vi "PJ1_ui-commu_1 -test.vi"() -> ()   [LabVIEW 2024]
uses:
  <vilib>/express/express analysis/Spectral/XNode/ExpressSpectralMeasurementsBlockNode.xnode
  <vilib>/express/express analysis/Spectral/Block/exnSpectralBlock spectral measurements PSD poly.vi
  <vilib>/express/express analysis/Spectral/Block/exnSpectralBlock spectral measurements PSD DDT.vi
  contron/Control 6.ctl
  contron/Control 7.ctl
  contron/Control 8.ctl
  <vilib>/picture/picture.llb/imagedata.ctl
  contol_vr 23/Control 9.ctl
  contol_vr 23/Control 3.ctl
  contol_vr 23/Control 4.ctl
  contol_vr 23/6.ctl
  contol_vr 23/66.ctl
  contron/Control 5.ctl
panel:
  out "Clear4":bool
  out "Clear 3":bool
  out "Clear2":bool
  out "check":bool
  out "Clear1":bool
  out "com":bool
  out "call":bool
  out "ele":bool
  in  "Baseline":bool
  out "555":bool
  out "6 HZ 2":bool
  out "image data":T1
  out "7 HZ":bool
  in  "Upper Cut-Off":dbl=40.0
  out "PSD":dynamicdata(graph)
  out "PSD MAX":dbl
  out "Index ที่มากที่สุด":i32
  out "max value":dbl
  out "B 18+1":dbl
  out "N 18+1":dbl
  in  "Aj 18+1":dbl
  out "B 18+1":dbl
  out "PSD 18+1":dbl
  out "B 18":dbl
  out "N 18":dbl
  in  "Aj 18":dbl
  out "B 18":dbl
  out "PSD 18":dbl
  out "B 18-1":dbl
  out "N 18-1":dbl
  in  "Aj 18-1":dbl
  out "B 18-1":dbl
  out "PSD 18-1":dbl
  out "9 Hz":dbl[](array[numeric])
  out "Max Index 9":i32
  out "PSD max 9":dbl
  out "PSD 9-1":dbl
  out "B 9-1":dbl
  in  "Aj 9-1":dbl
  out "N 9-1":dbl
  out "B 9-1":dbl
  out "PSD 9":dbl
  out "B 9":dbl
  in  "Aj 9":dbl
  out "N 9":dbl
  out "B 9":dbl
  out "PSD 9+1":dbl
  out "B 9+1":dbl
  in  "Aj 9+1":dbl
  out "N 9+1":dbl
  out "B 9+1":dbl
  out "8 Hz":dbl[](array[numeric])
  out "Max Index 8":i32
  out "PSD max 8":dbl
  out "B 16+1":dbl
  out "N 16+1":dbl
  in  "Aj  16+1":dbl
  out "B 16+1":dbl
  out "PSD  16+1":dbl
  out "B 16":dbl
  out "N  16":dbl
  in  "Aj  16":dbl
  out "B 16":dbl
  out "PSD  16":dbl
  out "B 16-1":dbl
  out "N  16-1":dbl
  in  "Aj   16-1":dbl
  out "B   16-1":dbl
  out "PSD 16-1":dbl
  out "B 8+1":dbl
  out "N 8+1":dbl
  in  "Aj  8+1":dbl
  out "B  8+1":dbl
  out "PSD 8+1":dbl
  out "B 8":dbl
  out "N  8":dbl
  in  "Aj  8":dbl
  out "B  8":dbl
  out "PSD 8":dbl
  out "B 8-1":dbl
  out "N  8-1":dbl
  in  "Aj  8-1":dbl
  out "B  8-1":dbl
  out "PSD 8-1":dbl
  out "PSD 14+1":dbl
  out "B 14+1":dbl
  in  "Aj 14+1":dbl
  out "N 14+1":dbl
  out "B 14+1":dbl
  out "PSD 14":dbl
  out "B 14":dbl
  in  "Aj 14":dbl
  out "N 14":dbl
  out "B 14":dbl
  out "PSD 14-1":dbl
  out "B 14-1":dbl
  in  "Aj 14-1":dbl
  out "N 14-1":dbl
  out "B 14-1":dbl
  out "PSD7+1":dbl
  out "B7+1":dbl
  in  "Aj7+1":dbl
  out "N7+1":dbl
  out "B7+1":dbl
  out "PSD 7":dbl
  out "B 7":dbl
  in  "Aj 7":dbl
  out "N7":dbl
  out "B7":dbl
  out "7 Hz":dbl[](array[numeric])
  out "Max Index 7":i32
  out "PSD max 7":dbl
  out "PSD 7-1":dbl
  out "B 7-1":dbl
  in  "Aj 7-1":dbl
  out "N7-1":dbl
  out "B7-1":dbl
  out "B12-1":dbl
  out "N12-1":dbl
  in  "Aj 12-1":dbl
  out "B 12-1":dbl
  out "PSD 12-1":dbl
  out "B12":dbl
  out "N12":dbl
  in  "Aj 12":dbl
  out "B12":dbl
  out "PSD 12":dbl
  out "B12+1":dbl
  out "N12+1":dbl
  in  "Aj 12+1":dbl
  out "B 12+1":dbl
  out "PSD 12+1":dbl
  out "B6+1":dbl
  out "N6+1":dbl
  in  "Aj 6+1":dbl
  out "B 6+1":dbl
  out "PSD 6+1":dbl
  out "B6":dbl
  out "N6":dbl
  in  "Aj 6":dbl
  out "B6":dbl
  out "PSD 6":dbl
  out "PSD 6-1":dbl
  out "6 Hz":dbl[](array[numeric])
  out "Max Index 6":i32
  out "PSD max 6":dbl
  out "B 6-1":dbl
  in  "Aj 6-1":dbl
  out "N6-1":dbl
  out "B6-1":dbl
  out "appended array":dbl[][](array[numeric])
  out "Filtered Signal":dynamicdata(graph)
  in  "Lower Cut-Off":dbl=1.0
  out "data":dynamicdata(graph) caption="Raw Data"
  in  "number of samples":i32=1000
  in  "rate":dbl=200.0 min=200.0 max=200.0
  out "?":bool
  out "?":bool
  out "?":bool
  out "?":bool
  out "?":bool
  out "?":bool
  out "?":bool
  out "?":bool
  out "?":bool
  out "?":bool
  out "?":bool=TRUE
  out "?":bool=TRUE
  out "?":bool=TRUE
  out "?":bool=TRUE
  out "?":bool=TRUE
  out "?":bool=TRUE
  out "?":bool=TRUE
  out "?":bool=TRUE
  out "?":bool=TRUE
  out "?":bool=TRUE
  out "?":bool
  out "?":bool
  out "?":bool
  out "?":bool
  out "?":bool
  out "?":bool
  out "?":bool
  out "?":bool
  out "?":bool
  out "?":bool
  out "?":bool=TRUE
  out "?":bool=TRUE
  out "?":bool=TRUE
  out "?":bool=TRUE
  out "?":bool=TRUE
  out "?":bool=TRUE
  out "?":bool=TRUE
  out "?":bool=TRUE
  out "?":bool=TRUE
  out "?":bool=TRUE
  out "?":bool
  out "?":bool
  out "?":bool
  out "?":bool
  out "?":bool
  out "?":bool
  out "?":bool
  out "?":bool
  out "?":bool
  out "?":bool
  out "?":bool=TRUE
  out "?":bool=TRUE
  out "?":bool=TRUE
  out "?":bool=TRUE
  out "?":bool=TRUE
  out "?":bool=TRUE
  out "?":bool=TRUE
  out "?":bool=TRUE
  out "?":bool=TRUE
  out "?":bool=TRUE
  out "?":bool
  out "?":bool
  out "?":bool
  out "?":bool
  out "?":bool
  out "?":bool
  out "?":bool
  out "?":bool
  out "?":bool
  out "?":bool
  out "?":bool=TRUE
  out "?":bool=TRUE
  out "?":bool=TRUE
  out "?":bool=TRUE
  out "?":bool=TRUE
  out "?":bool=TRUE
  out "?":bool=TRUE
  out "?":bool=TRUE
  out "?":bool=TRUE
  out "?":bool=TRUE
  out "9 HZ":bool
  out "8 HZ":bool
  in  "Tab Control":T2(tab)
  out "Emotion 7":bool
  out "Emotion 6":bool
  out "Emotion 5":bool
  out "Emotion 4":bool
  out "ele":T3
  out "Emer":bool
  out "call":T4
  out "commu":T5
  out "Activity":bool
  out "8-2":bool
  out "cummu_back":bool
  out "cummu_2":bool
  out "cummu_1":bool
  out "Emotion":bool
  out "ACC":T6
  out "back_page2":T7
  in  "send":bool
  out "call_back":bool
  out "call_3":bool
  out "call_back":bool
  out "call_2":bool
  out "call_1":bool
  out "1 3":bool
  out "1 2":T8
  out "1":bool
  out "String 2":string
  in  "SOS CALLING":bool
  in  "Search Button 2":bool
  out "ele_back":bool
  out "ele_3":bool
  out "ele_2":bool
  out "ele_1":bool
  out "ele_2":bool
  out "ele_3":bool
  out "ele_1":bool
  out "BACK_Page4":bool
  out "BACK_page5":bool
  out "Emotion 3":bool
  out "Emotion 2":bool
  in  "BACK_Page5":bool=TRUE
  in  "Button 3":bool=TRUE
  in  "Button 2":bool=TRUE
  in  "Button 1":bool=TRUE
  out "Emotion 1":bool
  out "Emotion 11":bool
  in  "BACK_Page6":T9
  out "Emotion 10":bool
  out "Emotion 9":bool
  out "Emotion 8":bool
  in  "Activity 1":path
  out "new picture":picture
  in  "Activity 2":path
  in  "Activity 3":path
  out "new picture 2":picture
  out "new picture 3":picture
  out "Emotion 19":bool
  out "Emotion 18":bool
  out "Emotion 17":bool
  out "Emotion 16":bool
  out "new picture 7":picture
  in  "AAC13":path
  in  "Massage Send 3":string
  out "new picture 6":picture
  in  "AAC1 2":path
  in  "Massage Send 2":string
  out "new picture 5":picture
  in  "AAC1":path
  in  "BACK_Page7":bool
  in  "Massage Send 2":string
  out "Message Display":string
  in  "send 3":bool
  in  "Message Send":string
  in  "Clearpage 2":bool
  in  "Text3":T10
  in  "Text2":T11
  in  "Text1":bool
  in  "send 2":bool
  # "MENU"
  # "COMMUNICATION"
  # "SOS CALLING"
  # "Tel."
  # "ELECTRICAL DEVICES"
  # "EMOTIONS"
  # "ACTIVITIES"
  # "AAC"
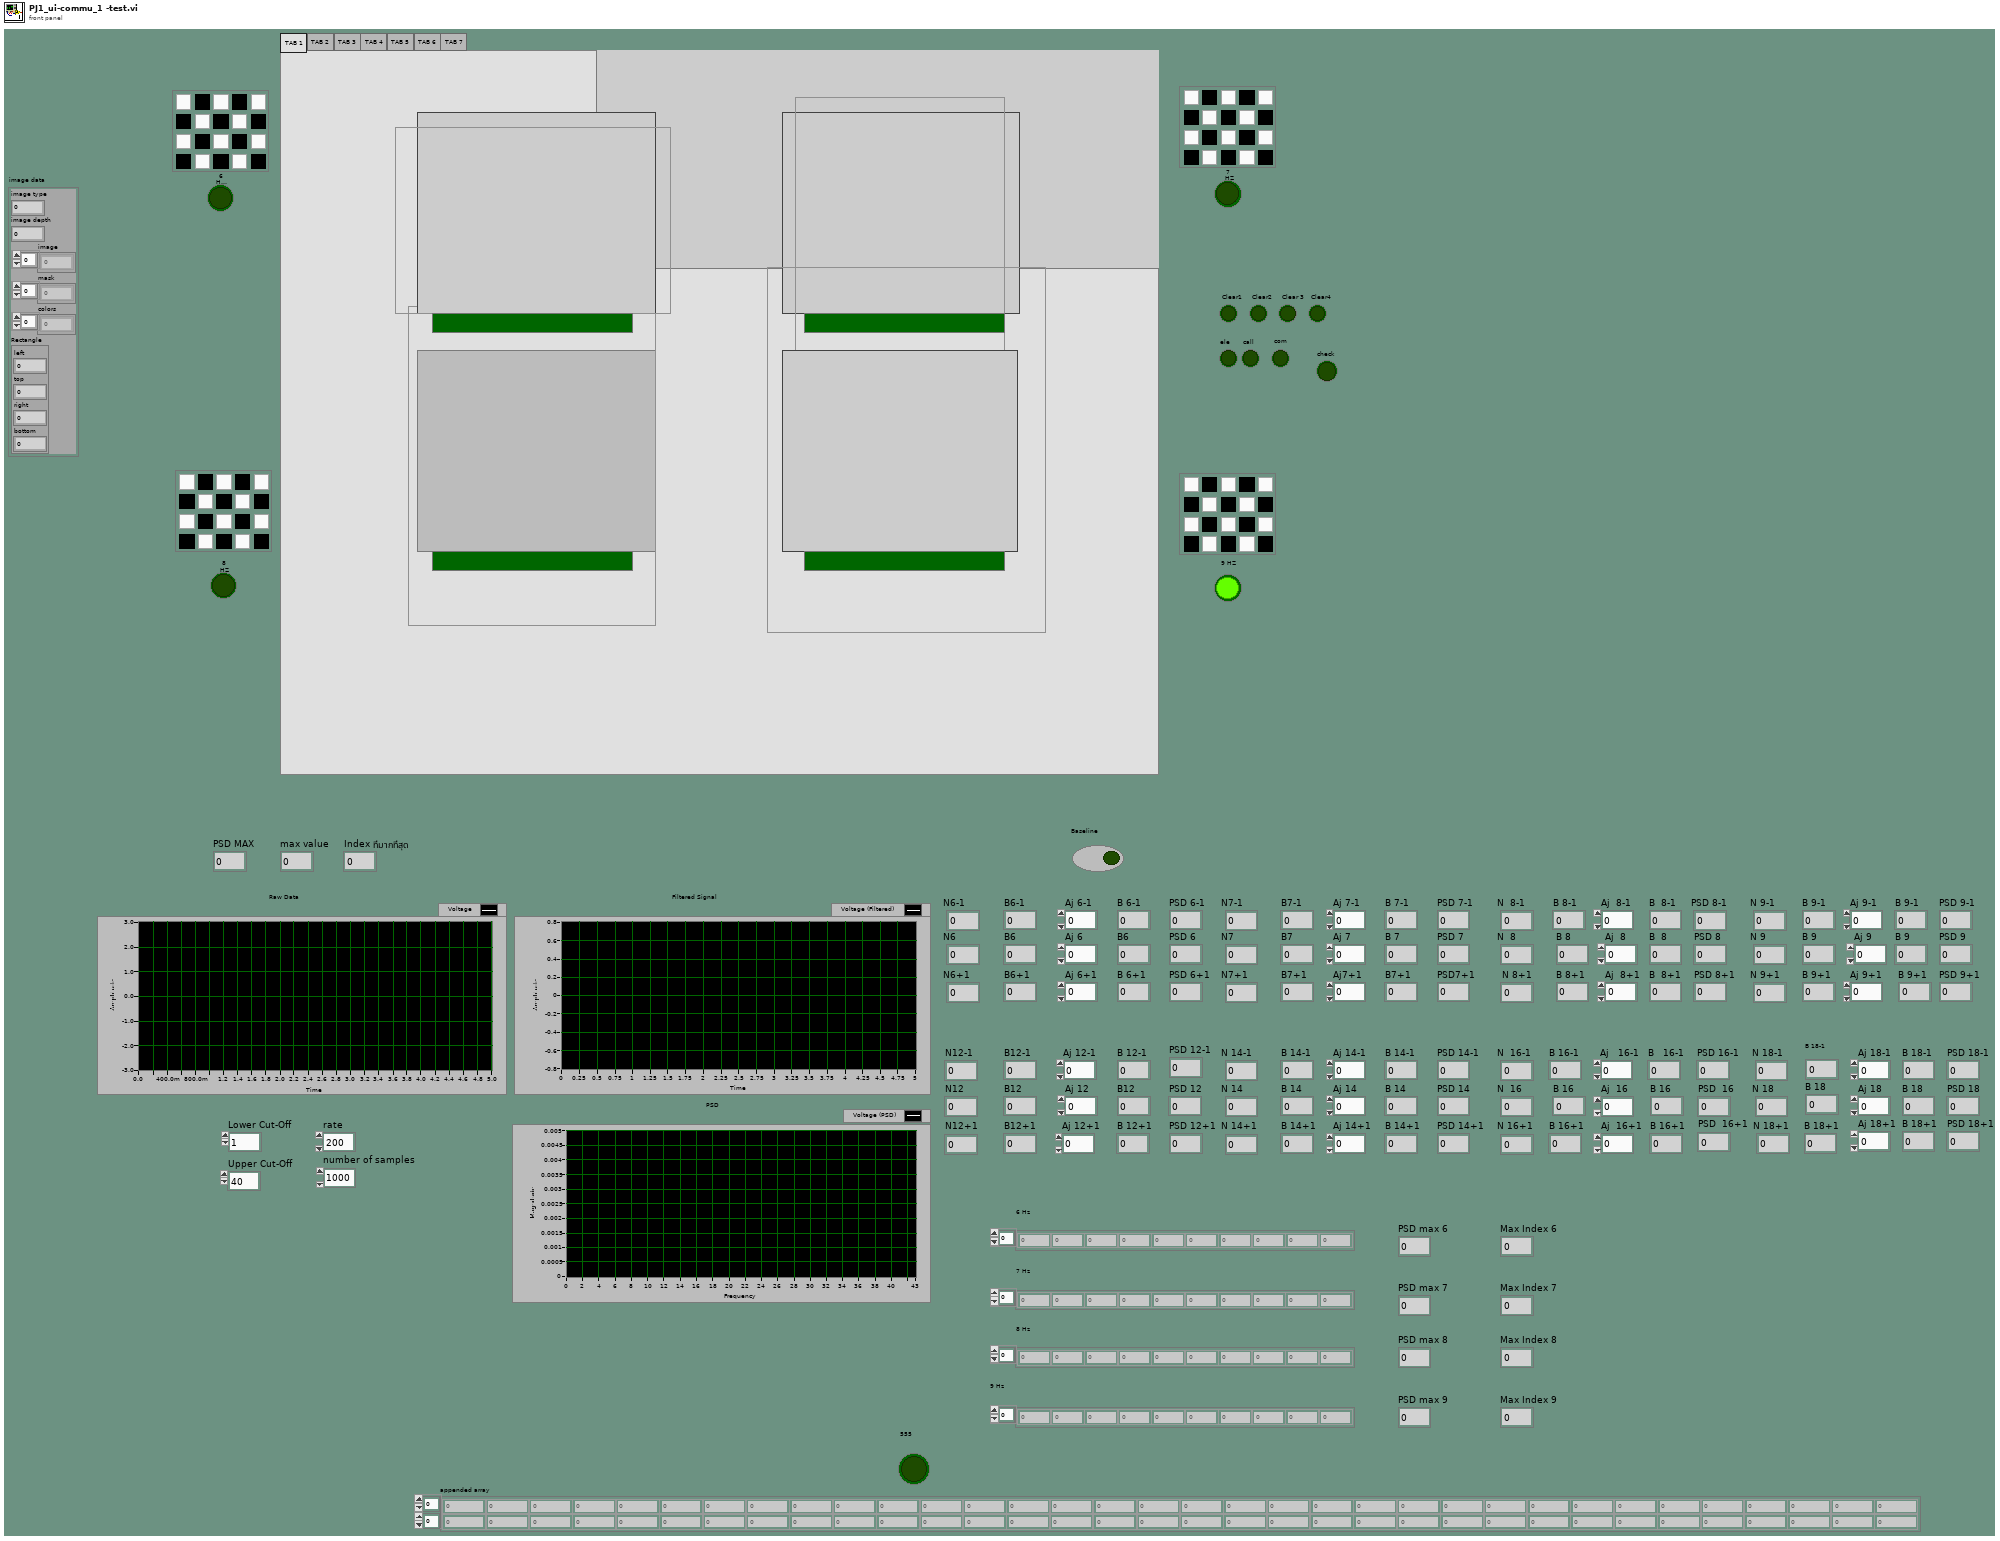
[diagram p1: front panel]
types:
  T1 = typedef "imagedata.ctl" = cluster{"image type":i32, "image depth":i32, "image":u8[], "mask":u8[], "colors":u32[], "Rectangle":cluster{"left":i16, "top":i16, "right":i16, "bottom":i16}}
  T2 = enum32{"TAB 1", "TAB 2", "TAB 3", "TAB 4", "TAB 5", "TAB 6", "TAB 7"}
  T3 = typedef "Control 5.ctl" = bool
  T4 = typedef "Control 6.ctl" = bool
  T5 = typedef "Control 7.ctl" = bool
  T6 = typedef "6.ctl" = bool
  T7 = typedef "66.ctl" = bool
  T8 = typedef "Control 8.ctl" = bool
  T9 = typedef "Control 9.ctl" = bool
  T10 = typedef "Control 4.ctl" = bool
  T11 = typedef "Control 3.ctl" = bool
  T12 = cluster{"averaging mode":u16, "weighting mode":u16, "number of averages":u32}
  T13 = cluster{"dB On (F)":bool, "unwrap phase (F)":bool, "convert to degree (F)":bool}
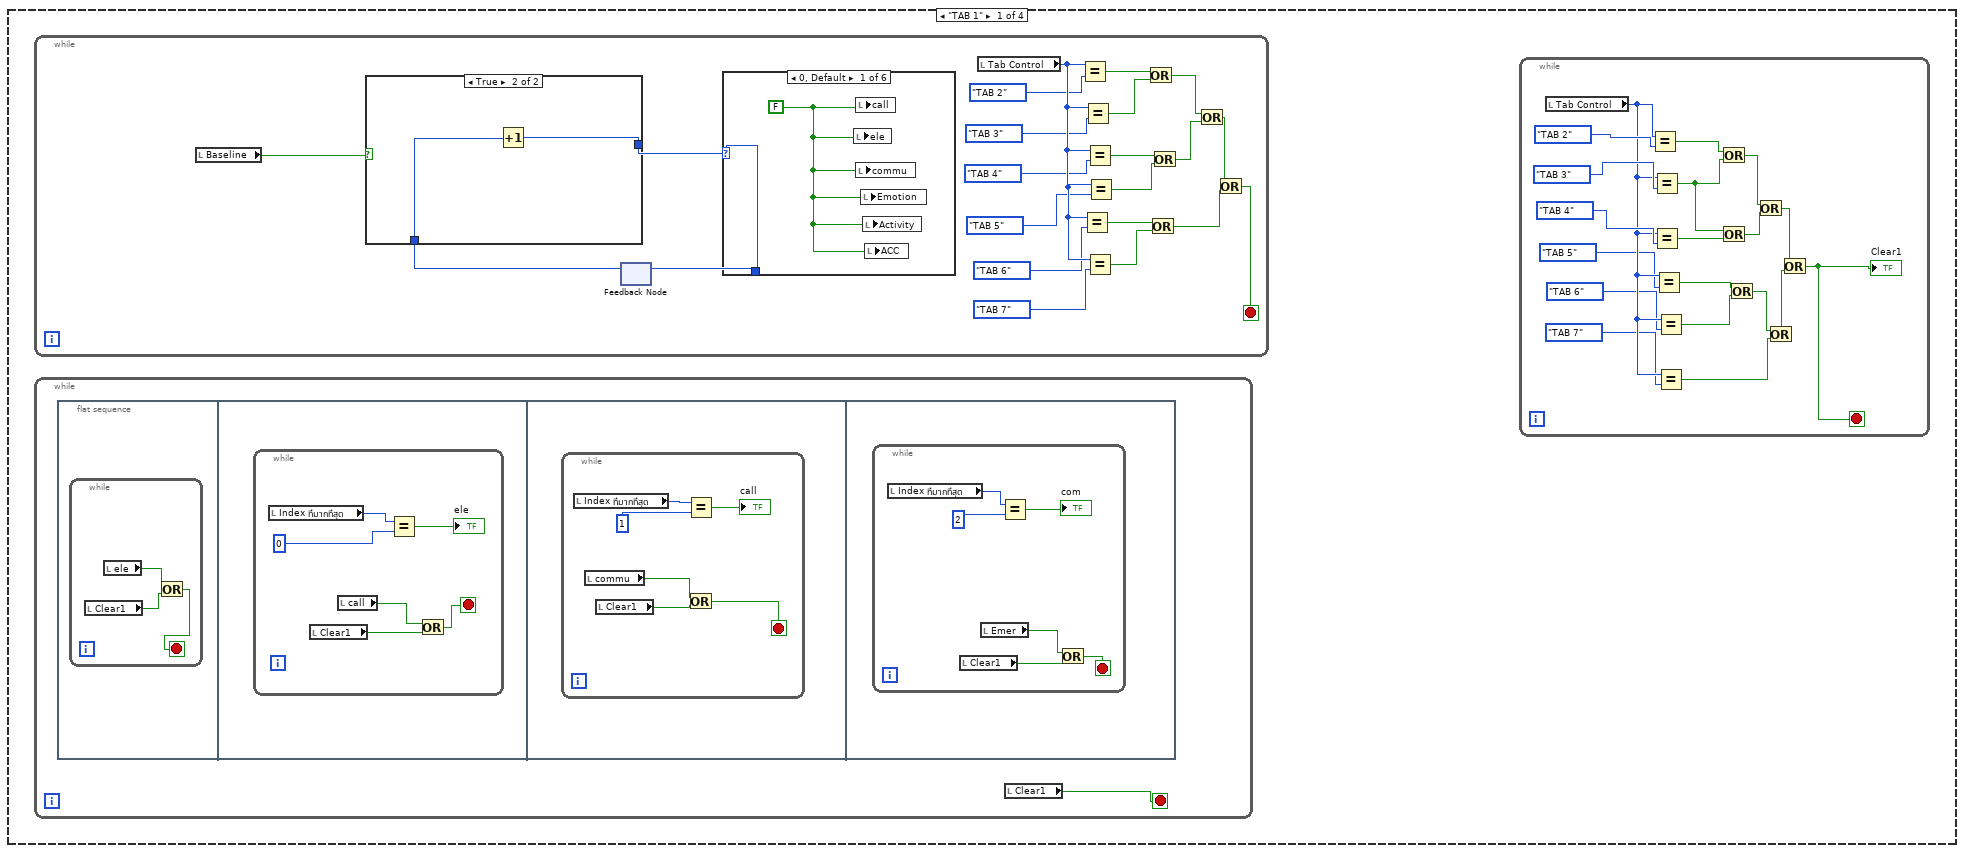
[diagram p2: hidden frame]
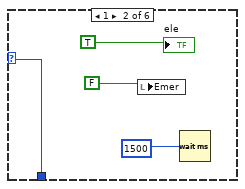
[diagram p3: hidden frame]
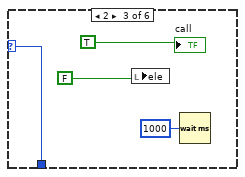
[diagram p4: hidden frame]
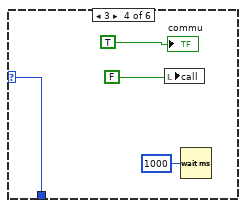
[diagram p5: hidden frame]
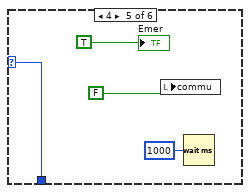
[diagram p6: hidden frame]
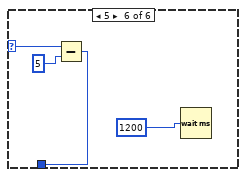
[diagram p7: hidden frame]
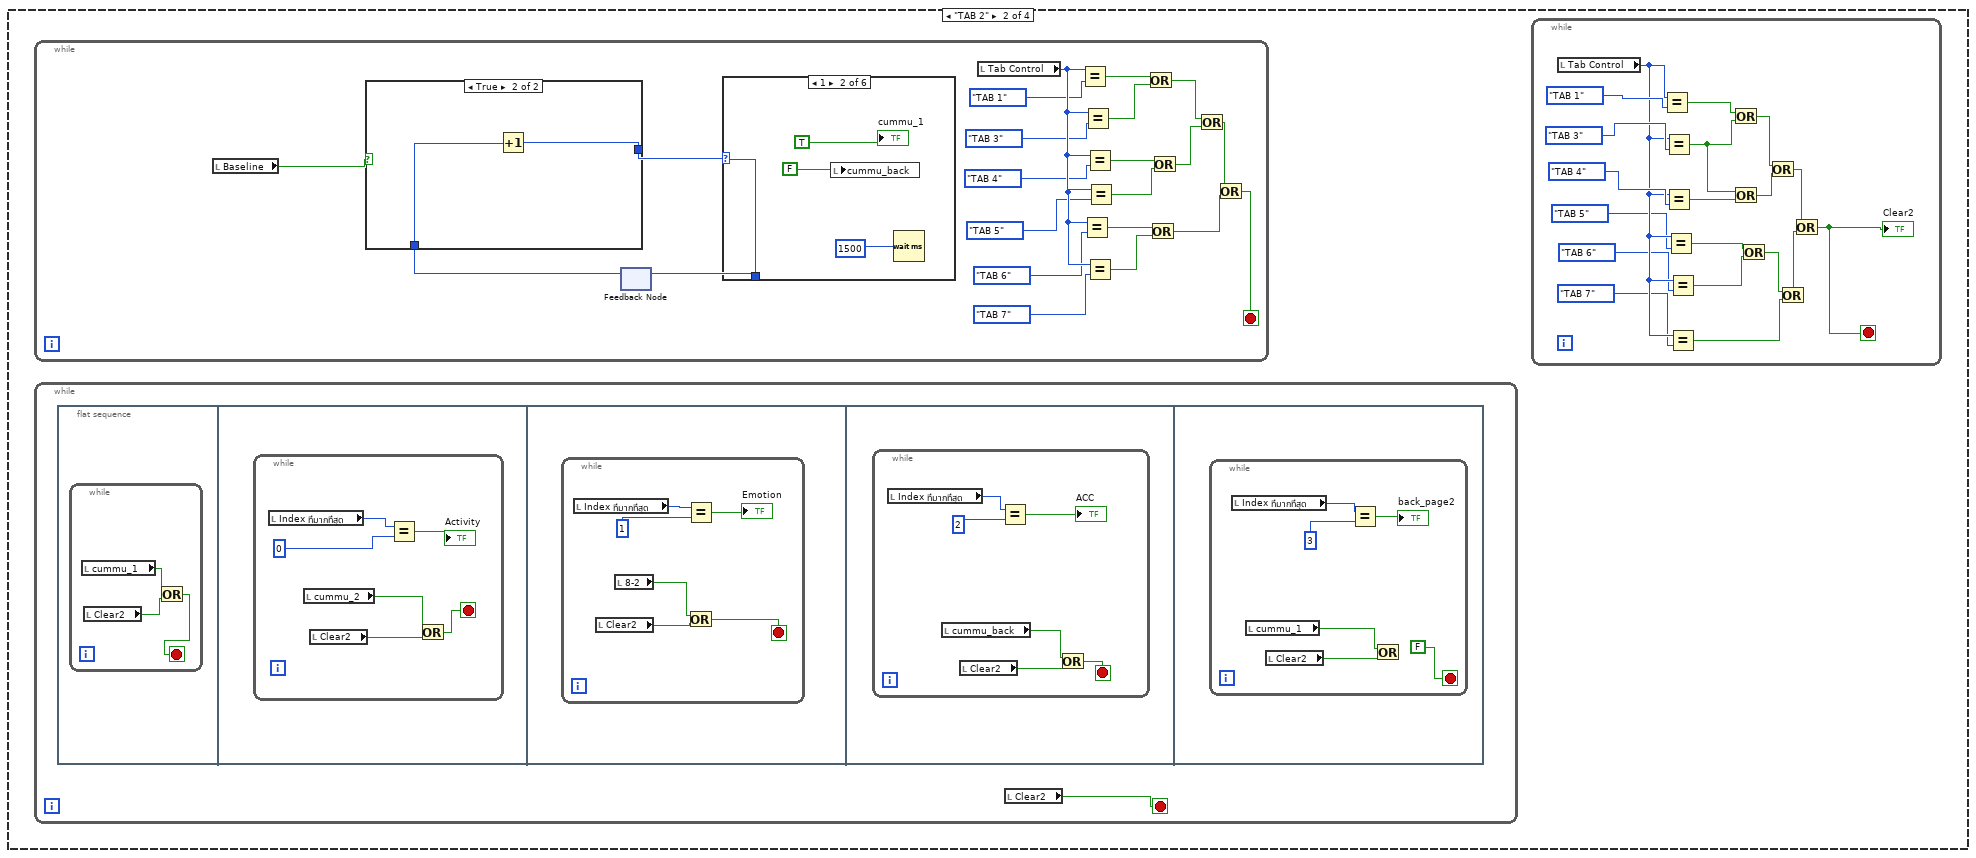
[diagram p9: hidden frame]
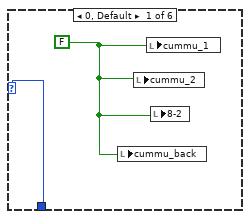
[diagram p10: hidden frame]
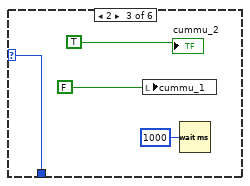
[diagram p11: hidden frame]
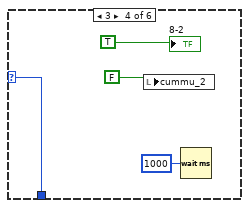
[diagram p12: hidden frame]
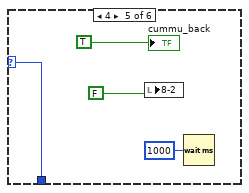
[diagram p13: hidden frame]
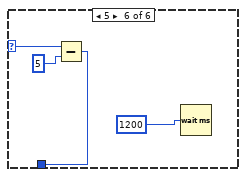
[diagram p14: hidden frame]
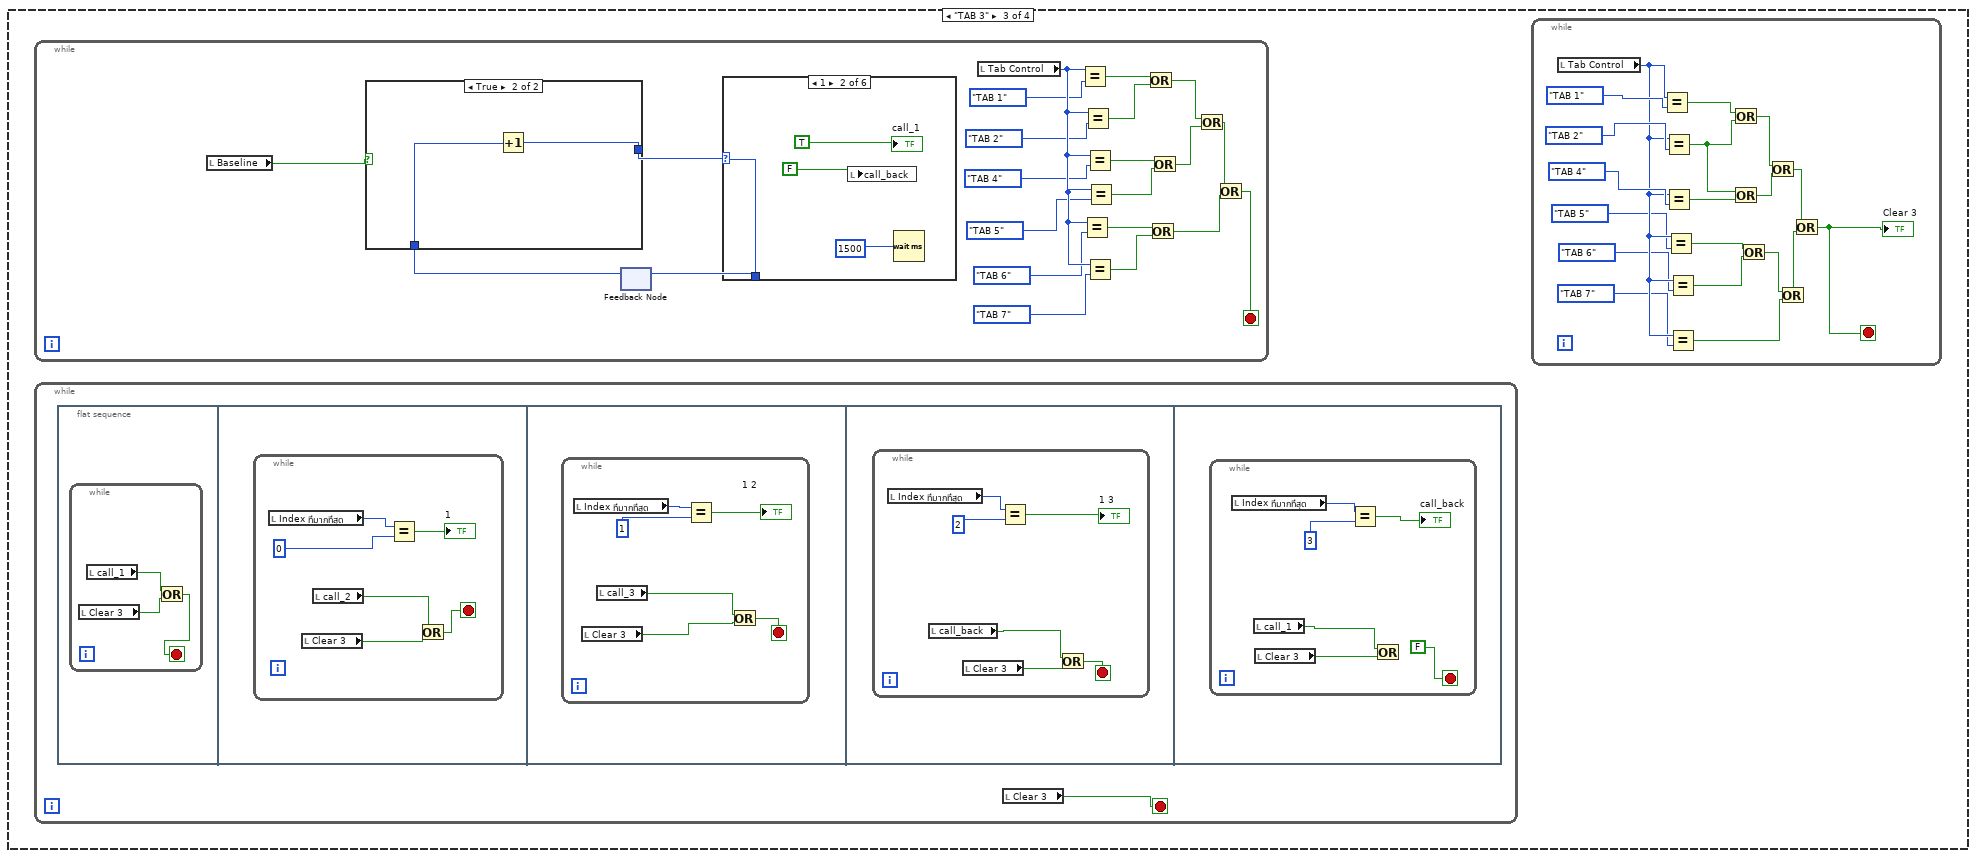
[diagram p16: hidden frame]
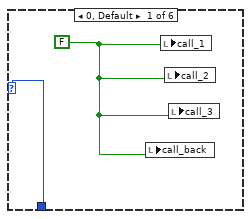
[diagram p17: hidden frame]
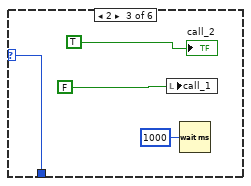
[diagram p18: hidden frame]
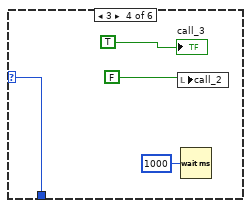
[diagram p19: hidden frame]
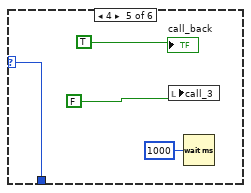
[diagram p20: hidden frame]
diagram:
  n1 = while {
    shift-right: [w17] -> _
    shift-left: "" -> [w19]
    stop <- FALSE stop-if-true
    n2 = event shown="[3] \"call_back\": Value Change" {
      selector: _ -> [_ _ _ _]
      dyn-events: _ -> [_ _ _ _]
      timeout: _ -> [_ _ _ _]
      tunnel: w19 -> [_ _ _ _]
      tunnel: ["0622436287" "1669" " 0937529340" _] -> w17
      event Value Change {
        n3 = event-data() -> ()  [unwired: 1 in, 6 out]
      }
      event "1": Value Change {
        n4 = event-data() -> ()  [unwired: 1 in, 6 out]
      }
      event "1 3": Value Change {
        n5 = event-data() -> ()  [unwired: 1 in, 6 out]
      }
      event "call_back": Value Change {
        n6 = event-data() -> ()  [unwired: 1 in, 6 out]
        n7 = local write "Tab Control"(enum32{"TAB 1", "TAB 2", "TAB 3", "TAB 4"}."TAB 1" ("Tab Control")) -> ()
      }
    }
    "String 2" <- w17
  }
  n8 = while {
    stop <- FALSE stop-if-true
    n9 = while {
      stop <- FALSE stop-if-true
      n10 = while {
        stop <- FALSE stop-if-true
        w63 = 83.3333
        # "6 HZ"
        n11 = for {
          N: 2 -> [_]
          tunnel: w63 -> [w67]
          i -> [w69]
          n12 = Wait (ms)(milliseconds to wait=w67) -> ()  [unwired: 1 out]
          n13 = Equal?(x=0, y=w69) -> (x = y?=→"?" →"?" →"?" →"?" →"?" →"?" →"?" →"?" →"?" →"?":bool)
        }
        n14 = for {
          N: 2 -> [_]
          tunnel: w63 -> [w71]
          i -> [w72]
          n15 = Wait (ms)(milliseconds to wait=w71) -> ()  [unwired: 1 out]
          n16 = Equal?(x=1, y=w72) -> (x = y?=→"?" →"?" →"?" →"?" →"?" →"?" →"?" →"?" →"?" →"?":bool)
        }
      }
      n17 = while {
        stop <- FALSE stop-if-true
        w51 = 71.428571
        # "7 HZ"
        n18 = for {
          N: 2 -> [_]
          tunnel: w51 -> [w55]
          i -> [w57]
          n19 = Wait (ms)(milliseconds to wait=w55) -> ()  [unwired: 1 out]
          n20 = Equal?(x=0, y=w57) -> (x = y?=→"?" →"?" →"?" →"?" →"?" →"?" →"?" →"?" →"?" →"?":bool)
        }
        n21 = for {
          N: 2 -> [_]
          tunnel: w51 -> [w59]
          i -> [w60]
          n22 = Wait (ms)(milliseconds to wait=w59) -> ()  [unwired: 1 out]
          n23 = Equal?(x=1, y=w60) -> (x = y?=→"?" →"?" →"?" →"?" →"?" →"?" →"?" →"?" →"?" →"?":bool)
        }
      }
      n24 = while {
        stop <- FALSE stop-if-true
        w39 = 62.5
        # "8 HZ"
        n25 = for {
          N: 2 -> [_]
          tunnel: w39 -> [w43]
          i -> [w45]
          n26 = Wait (ms)(milliseconds to wait=w43) -> ()  [unwired: 1 out]
          n27 = Equal?(x=0, y=w45) -> (x = y?=→"?" →"?" →"?" →"?" →"?" →"?" →"?" →"?" →"?" →"?":bool)
        }
        n28 = for {
          N: 2 -> [_]
          tunnel: w39 -> [w47]
          i -> [w48]
          n29 = Wait (ms)(milliseconds to wait=w47) -> ()  [unwired: 1 out]
          n30 = Equal?(x=1, y=w48) -> (x = y?=→"?" →"?" →"?" →"?" →"?" →"?" →"?" →"?" →"?" →"?":bool)
        }
      }
      n31 = while {
        stop <- FALSE stop-if-true
        w27 = 55.5555
        # "9 HZ"
        n32 = for {
          N: 2 -> [_]
          tunnel: w27 -> [w31]
          i -> [w33]
          n33 = Wait (ms)(milliseconds to wait=w31) -> ()  [unwired: 1 out]
          n34 = Equal?(x=0, y=w33) -> (x = y?=→"?" →"?" →"?" →"?" →"?" →"?" →"?" →"?" →"?" →"?":bool)
        }
        n35 = for {
          N: 2 -> [_]
          tunnel: w27 -> [w35]
          i -> [w36]
          n36 = Wait (ms)(milliseconds to wait=w35) -> ()  [unwired: 1 out]
          n37 = Equal?(x=1, y=w36) -> (x = y?=→"?" →"?" →"?" →"?" →"?" →"?" →"?" →"?" →"?" →"?":bool)
        }
      }
    }
  }
  n38 = while {
    stop <- FALSE stop-if-true
    n39 = call "DAQ Assistant2"("rate"="rate", "number of samples"="number of samples") -> ("data"=w78:dynamicdata)  [unwired: 15 in, 2 out]
    "data" <- w78
    n40 = Divide(x="rate", y="number of samples") -> (x/y=w165:dbl)
    n41 = call "Filter"("Lower Cut-Off"="Lower Cut-Off", "Upper Cut-Off"="Upper Cut-Off", "Signal"=w78) -> ("Filtered Signal"=w79:dynamicdata)  [unwired: 7 in, 1 out]
    "Filtered Signal" <- w79
    n42 = Divide(x=8.0, y=w165) -> (x/y=w265:dbl)
    n43 = Divide(x=16.0, y=w165) -> (x/y=w217:dbl)
    n44 = Divide(x=14.0, y=w165) -> (x/y=w290:dbl)
    n45 = Divide(x=18.0, y=w165) -> (x/y=w140:dbl)
    n46 = xnode "Spectral Measurements"("Signals"=w79) -> ("PSD"=w105:dynamicdata)  [unwired: 1 in, 1 out]
    "PSD" <- w105
    n47 = Divide(x=9.0, y=w165) -> (x/y=w183:dbl)
    n48 = Divide(x=7.0, y=w165) -> (x/y=w307:dbl)
    n49 = Divide(x=12.0, y=w165) -> (x/y=w376:dbl)
    n50 = Divide(x=6.0, y=w165) -> (x/y=w425:dbl)
    n51 = call "Convert from Dynamic Data"("Dynamic Data Type"=w105) -> ("Array"=w455:dbl[])  [unwired: 3 in]
    n52 = Decrement(x=w183) -> (x-1=w214:dbl)
    n53 = Increment(x=w183) -> (x+1=w182:dbl)
    n54 = Increment(x=w140) -> (x+1=w129:dbl)
    n55 = Decrement(x=w140) -> (x-1=w154:dbl)
    n56 = Decrement(x=w290) -> (x-1=w319:dbl)
    n57 = Increment(x=w265) -> (x+1=w255:dbl)
    n58 = Decrement(x=w217) -> (x-1=w240:dbl)
    n59 = Decrement(x=w425) -> (x-1=w438:dbl)
    n60 = Decrement(x=w307) -> (x-1=w348:dbl)
    "PSD 7-1" <- w348
    n61 = Increment(x=w307) -> (x+1=w333:dbl)
    n62 = Decrement(x=w265) -> (x-1=w278:dbl)
    n63 = Increment(x=w217) -> (x+1=w216:dbl)
    n64 = Increment(x=w425) -> (x+1=w414:dbl)
    n65 = Increment(x=w290) -> (x+1=w296:dbl)
    n66 = Decrement(x=w376) -> (x-1=w381:dbl)
    n67 = Increment(x=w376) -> (x+1=w375:dbl)
    n68 = Build Array(w455) -> (w130:dbl[][])
    "appended array" <- w130
    n69 = Index Array(array=w130, index (row)=0, index (col)=w240) -> (element=w251:dbl)
    "PSD 16-1" <- w251
    n70 = Index Array(array=w130, index (row)=0 ("disabled index (row)"), index (col)=w216) -> (element=w228:dbl)
    "PSD  16+1" <- w228
    n71 = Index Array(array=w130, index (row)=0 ("disabled index (row)"), index (col)=w217) -> (element=w230:dbl)
    "PSD  16" <- w230
    n72 = Index Array(array=w130, index (row)=0, index (col)=w296) -> (element=w297:dbl)
    "PSD 14+1" <- w297
    n73 = Index Array(array=w130, index (row)=0 ("disabled index (row)"), index (col)=w154) -> (element=w152:dbl)
    "PSD 18-1" <- w152
    n74 = Index Array(array=w130, index (row)=0, index (col)=w255) -> (element=w253:dbl)
    "PSD 8+1" <- w253
    n75 = Index Array(array=w130, index (row)=0 ("disabled index (row)"), index (col)=w129) -> (element=w126:dbl)
    "PSD 18+1" <- w126
    n76 = Index Array(array=w130, index (row)=0, index (col)=w182) -> (element=w171:dbl)
    "PSD 9-1" <- w171
    n77 = Index Array(array=w130, index (row)=0, index (col)=w265) -> (element=w276:dbl)
    "PSD 8" <- w276
    n78 = Index Array(array=w130, index (row)=0 ("disabled index (row)"), index (col)=w140) -> (element=w141:dbl)
    "PSD 18" <- w141
    n79 = Index Array(array=w130, index (row)=0, index (col)=w278) -> (element=w277:dbl)
    "PSD 8-1" <- w277
    n80 = Index Array(array=w130, index (row)=0, index (col)=w183) -> (element=w184:dbl)
    "PSD 9" <- w184
    n81 = Index Array(array=w130, index (row)=0, index (col)=w214) -> (element=w195:dbl)
    "PSD 9+1" <- w195
    n82 = Index Array(array=w130, index (row)=0, index (col)=w319) -> (element=w321:dbl)
    "PSD 14-1" <- w321
    n83 = Index Array(array=w130, index (row)=0, index (col)=w290) -> (element=w308:dbl)
    "PSD 14" <- w308
    n84 = Index Array(array=w130, index (row)=0, index (col)=w348) -> ()  [unwired: 1 out]
    n85 = Index Array(array=w130, index (row)=0 ("disabled index (row)"), index (col)=w307) -> (element=w345:dbl)
    "PSD 7" <- w345
    n86 = Index Array(array=w130, index (row)=0, index (col)=w333) -> (element=w334:dbl)
    "PSD7+1" <- w334
    n87 = Index Array(array=w130, index (row)=0 ("disabled index (row)"), index (col)=w414) -> (element=w412:dbl)
    "PSD 6+1" <- w412
    n88 = Index Array(array=w130, index (row)=0, index (col)=w381) -> (element=w380:dbl)
    "PSD 12-1" <- w380
    n89 = Index Array(array=w130, index (row)=0 ("disabled index (row)"), index (col)=w376) -> (element=w377:dbl)
    "PSD 12" <- w377
    n90 = Index Array(array=w130, index (row)=0 ("disabled index (row)"), index (col)=w375) -> (element=w373:dbl)
    "PSD 12+1" <- w373
    n91 = Index Array(array=w130, index (row)=0, index (col)=w425) -> (element=w426:dbl)
    "PSD 6" <- w426
    n92 = Index Array(array=w130, index (row)=0, index (col)=w438) -> (element=w445:dbl)
    "PSD 6-1" <- w445
    n93 = feedback #1() -> (w81:dbl)  [unwired: 1 in]
    "B 18" <- w81
    n94 = case shown="False" "Baseline" {
      tunnel: w141 -> [_ w466]
      tunnel: [w465 w466] -> w143
      tunnel: w81 -> [w465 _]
      frame False {
      }
      frame True {
      }
    }
    n95 = feedback-in #1(w143) -> ()
    n96 = feedback #2() -> (w82:dbl)  [unwired: 1 in]
    "B 18-1" <- w82
    n97 = case shown="False" "Baseline" {
      tunnel: w152 -> [_ w470]
      tunnel: [w469 w470] -> w163
      tunnel: w82 -> [w469 _]
      frame False {
      }
      frame True {
      }
    }
    n98 = feedback-in #2(w163) -> ()
    n99 = feedback #3() -> (w80:dbl)  [unwired: 1 in]
    "B 18+1" <- w80
    n100 = case shown="False" "Baseline" {
      tunnel: w126 -> [_ w462]
      tunnel: [w461 w462] -> w139
      tunnel: w80 -> [w461 _]
      frame False {
      }
      frame True {
      }
    }
    n101 = feedback-in #3(w139) -> ()
    n102 = feedback #4() -> (w88:dbl)  [unwired: 1 in]
    "B 16-1" <- w88
    n103 = case shown="True" "Baseline" {
      tunnel: w251 -> [_ w494]
      tunnel: [w493 w494] -> w241
      tunnel: w88 -> [w493 _]
      frame False {
      }
      frame True {
      }
    }
    n104 = feedback-in #4(w241) -> ()
    n105 = feedback #5() -> (w86:dbl)  [unwired: 1 in]
    "B 16+1" <- w86
    n106 = case shown="True" "Baseline" {
      tunnel: w228 -> [_ w486]
      tunnel: [w485 w486] -> w219
      tunnel: w86 -> [w485 _]
      frame False {
      }
      frame True {
      }
    }
    n107 = feedback-in #5(w219) -> ()
    n108 = feedback #6() -> (w87:dbl)  [unwired: 1 in]
    "B 16" <- w87
    n109 = case shown="True" "Baseline" {
      tunnel: w230 -> [_ w490]
      tunnel: [w489 w490] -> w239
      tunnel: w87 -> [w489 _]
      frame False {
      }
      frame True {
      }
    }
    n110 = feedback-in #6(w239) -> ()
    n111 = feedback #7() -> (w89:dbl)  [unwired: 1 in]
    "B 8+1" <- w89
    n112 = case shown="True" "Baseline" {
      tunnel: w253 -> [_ w498]
      tunnel: [w497 w498] -> w264
      tunnel: w89 -> [w497 _]
      frame False {
      }
      frame True {
      }
    }
    n113 = feedback-in #7(w264) -> ()
    n114 = feedback #8() -> (w92:dbl)  [unwired: 1 in]
    "B 14+1" <- w92
    n115 = case shown="True" "Baseline" {
      tunnel: w297 -> [_ w510]
      tunnel: [w509 w510] -> w298
      tunnel: w92 -> [w509 _]
      frame False {
      }
      frame True {
      }
    }
    n116 = feedback-in #8(w298) -> ()
    n117 = feedback #9() -> (w90:dbl)  [unwired: 1 in]
    "B 8" <- w90
    n118 = case shown="True" "Baseline" {
      tunnel: w276 -> [_ w502]
      tunnel: [w501 w502] -> w267
      tunnel: w90 -> [w501 _]
      frame False {
      }
      frame True {
      }
    }
    n119 = feedback-in #9(w267) -> ()
    n120 = feedback #10() -> (w84:dbl)  [unwired: 1 in]
    "B 9" <- w84
    n121 = case shown="False" "Baseline" {
      tunnel: w184 -> [_ w478]
      tunnel: [w477 w478] -> w185
      tunnel: w84 -> [w477 _]
      frame False {
      }
      frame True {
      }
    }
    n122 = feedback-in #10(w185) -> ()
    n123 = feedback #11() -> (w91:dbl)  [unwired: 1 in]
    "B 8-1" <- w91
    n124 = case shown="True" "Baseline" {
      tunnel: w277 -> [_ w506]
      tunnel: [w505 w506] -> w288
      tunnel: w91 -> [w505 _]
      frame False {
      }
      frame True {
      }
    }
    n125 = feedback-in #11(w288) -> ()
    n126 = feedback #12() -> (w85:dbl)  [unwired: 1 in]
    "B 9+1" <- w85
    n127 = case shown="True" "Baseline" {
      tunnel: w195 -> [_ w482]
      tunnel: [w481 w482] -> w196
      tunnel: w85 -> [w481 _]
      frame False {
      }
      frame True {
      }
    }
    n128 = feedback-in #12(w196) -> ()
    n129 = feedback #13() -> (w100:dbl)  [unwired: 1 in]
    "B12-1" <- w100
    n130 = case shown="True" "Baseline" {
      tunnel: w380 -> [_ w542]
      tunnel: [w541 w542] -> w392
      tunnel: w100 -> [w541 _]
      frame False {
      }
      frame True {
      }
    }
    n131 = feedback-in #13(w392) -> ()
    n132 = feedback #14() -> (w94:dbl)  [unwired: 1 in]
    "B 14-1" <- w94
    n133 = case shown="True" "Baseline" {
      tunnel: w321 -> [_ w518]
      tunnel: [w517 w518] -> w322
      tunnel: w94 -> [w517 _]
      frame False {
      }
      frame True {
      }
    }
    n134 = feedback-in #14(w322) -> ()
    n135 = feedback #15() -> (w83:dbl)  [unwired: 1 in]
    "B 9-1" <- w83
    n136 = case shown="False" "Baseline" {
      tunnel: w171 -> [_ w474]
      tunnel: [w473 w474] -> w172
      tunnel: w83 -> [w473 _]
      frame False {
      }
      frame True {
      }
    }
    n137 = feedback-in #15(w172) -> ()
    n138 = feedback #16() -> (w101:dbl)  [unwired: 1 in]
    "B6+1" <- w101
    n139 = case shown="True" "Baseline" {
      tunnel: w412 -> [_ w546]
      tunnel: [w545 w546] -> w415
      tunnel: w101 -> [w545 _]
      frame False {
      }
      frame True {
      }
    }
    n140 = feedback-in #16(w415) -> ()
    n141 = feedback #17() -> (w102:dbl)  [unwired: 1 in]
    "B6" <- w102
    n142 = case shown="True" "Baseline" {
      tunnel: w426 -> [_ w550]
      tunnel: [w549 w550] -> w436
      tunnel: w102 -> [w549 _]
      frame False {
      }
      frame True {
      }
    }
    n143 = feedback-in #17(w436) -> ()
    n144 = feedback #18() -> (w103:dbl)  [unwired: 1 in]
    "B6-1" <- w103
    n145 = case shown="False" "Baseline" {
      tunnel: w445 -> [_ w554]
      tunnel: [w553 w554] -> w437
      tunnel: w103 -> [w553 _]
      frame False {
      }
      frame True {
      }
    }
    n146 = feedback-in #18(w437) -> ()
    n147 = feedback #19() -> (w93:dbl)  [unwired: 1 in]
    "B 14" <- w93
    n148 = case shown="True" "Baseline" {
      tunnel: w308 -> [_ w514]
      tunnel: [w513 w514] -> w310
      tunnel: w93 -> [w513 _]
      frame False {
      }
      frame True {
      }
    }
    n149 = feedback-in #19(w310) -> ()
    n150 = feedback #20() -> (w98:dbl)  [unwired: 1 in]
    "B12+1" <- w98
    n151 = case shown="True" "Baseline" {
      tunnel: w373 -> [_ w534]
      tunnel: [w533 w534] -> w410
      tunnel: w98 -> [w533 _]
      frame False {
      }
      frame True {
      }
    }
    n152 = feedback-in #20(w410) -> ()
    n153 = Add(x=w81, y="Aj 18") -> (x+y=w147:dbl)
    "B 18" <- w147
    n154 = Add(x=w82, y="Aj 18-1") -> (x+y=w159:dbl)
    "B 18-1" <- w159
    n155 = Add(x=w80, y="Aj 18+1") -> (x+y=w135:dbl)
    "B 18+1" <- w135
    n156 = feedback #21() -> (w99:dbl)  [unwired: 1 in]
    "B12" <- w99
    n157 = case shown="True" "Baseline" {
      tunnel: w377 -> [_ w538]
      tunnel: [w537 w538] -> w393
      tunnel: w99 -> [w537 _]
      frame False {
      }
      frame True {
      }
    }
    n158 = feedback-in #21(w393) -> ()
    n159 = Add(x=w88, y="Aj   16-1") -> (x+y=w245:dbl)
    "B   16-1" <- w245
    n160 = Add(x=w86, y="Aj  16+1") -> (x+y=w223:dbl)
    "B 16+1" <- w223
    n161 = Add(x=w87, y="Aj  16") -> (x+y=w235:dbl)
    "B 16" <- w235
    n162 = Add(x=w89, y="Aj  8+1") -> (x+y=w260:dbl)
    "B  8+1" <- w260
    n163 = Add(x=w92, y="Aj 14+1") -> (x+y=w302:dbl)
    "B 14+1" <- w302
    n164 = Add(x=w90, y="Aj  8") -> (x+y=w271:dbl)
    "B  8" <- w271
    n165 = Add(x=w84, y="Aj 9") -> (x+y=w189:dbl)
    "B 9" <- w189
    n166 = Add(x=w91, y="Aj  8-1") -> (x+y=w284:dbl)
    "B  8-1" <- w284
    n167 = Add(x=w85, y="Aj 9+1") -> (x+y=w200:dbl)
    "B 9+1" <- w200
    n168 = Add(x=w100, y="Aj 12-1") -> (x+y=w388:dbl)
    "B 12-1" <- w388
    n169 = Add(x=w94, y="Aj 14-1") -> (x+y=w326:dbl)
    "B 14-1" <- w326
    n170 = Add(x=w83, y="Aj 9-1") -> (x+y=w176:dbl)
    "B 9-1" <- w176
    n171 = Multiply(x=w81, y=5.0) -> (x*y=w150:dbl)
    "N 18" <- w150
    n172 = Add(x=w101, y="Aj 6+1") -> (x+y=w419:dbl)
    "B 6+1" <- w419
    n173 = Multiply(x=w82, y=5.0) -> (x*y=w156:dbl)
    "N 18-1" <- w156
    n174 = Multiply(x=w80, y=5.0) -> (x*y=w132:dbl)
    "N 18+1" <- w132
    n175 = feedback #22() -> (w95:dbl)  [unwired: 1 in]
    "B7+1" <- w95
    n176 = case shown="True" "Baseline" {
      tunnel: w334 -> [_ w522]
      tunnel: [w521 w522] -> w336
      tunnel: w95 -> [w521 _]
      frame False {
      }
      frame True {
      }
    }
    n177 = feedback-in #22(w336) -> ()
    n178 = feedback #23() -> (w96:dbl)  [unwired: 1 in]
    "B7" <- w96
    n179 = case shown="True" "Baseline" {
      tunnel: w345 -> [_ w526]
      tunnel: [w525 w526] -> w349
      tunnel: w96 -> [w525 _]
      frame False {
      }
      frame True {
      }
    }
    n180 = feedback-in #23(w349) -> ()
    n181 = Multiply(x=w88, y=5.0) -> (x*y=w248:dbl)
    "N  16-1" <- w248
    n182 = Multiply(x=w86, y=5.0) -> (x*y=w226:dbl)
    "N 16+1" <- w226
    n183 = Multiply(x=w87, y=5.0) -> (x*y=w232:dbl)
    "N  16" <- w232
    n184 = Multiply(x=w89, y=5.0) -> (x*y=w257:dbl)
    "N 8+1" <- w257
    n185 = feedback #24() -> (w97:dbl)  [unwired: 1 in]
    "B7-1" <- w97
    n186 = case shown="True" "Baseline" {
      tunnel: w348 -> [_ w530]
      tunnel: [w529 w530] -> w362
      tunnel: w97 -> [w529 _]
      frame False {
      }
      frame True {
      }
    }
    n187 = feedback-in #24(w362) -> ()
    n188 = Add(x=w102, y="Aj 6") -> (x+y=w432:dbl)
    "B6" <- w432
    n189 = Add(x=w103, y="Aj 6-1") -> (x+y=w446:dbl)
    "B 6-1" <- w446
    n190 = Add(x=w93, y="Aj 14") -> (x+y=w314:dbl)
    "B 14" <- w314
    n191 = Multiply(x=w92, y=5.0) -> (x*y=w305:dbl)
    "N 14+1" <- w305
    n192 = Multiply(x=w90, y=5.0) -> (x*y=w274:dbl)
    "N  8" <- w274
    n193 = Multiply(x=w84, y=5.0) -> (x*y=w192:dbl)
    "N 9" <- w192
    n194 = Multiply(x=w91, y=5.0) -> (x*y=w281:dbl)
    "N  8-1" <- w281
    n195 = Multiply(x=w85, y=5.0) -> (x*y=w203:dbl)
    "N 9+1" <- w203
    n196 = Add(x=w98, y="Aj 12+1") -> (x+y=w406:dbl)
    "B 12+1" <- w406
    n197 = Multiply(x=w100, y=5.0) -> (x*y=w385:dbl)
    "N12-1" <- w385
    n198 = Multiply(x=w94, y=5.0) -> (x*y=w329:dbl)
    "N 14-1" <- w329
    n199 = Add(x=w99, y="Aj 12") -> (x+y=w397:dbl)
    "B12" <- w397
    n200 = Multiply(x=w83, y=5.0) -> (x*y=w179:dbl)
    "N 9-1" <- w179
    n201 = Multiply(x=w101, y=5.0) -> (x*y=w422:dbl)
    "N6+1" <- w422
    n202 = Greater?(x=w141, y=w147) -> (0:w148:bool)
    n203 = Greater?(x=w152, y=w159) -> (0:w158:bool)
    n204 = Greater?(x=w126, y=w135) -> (0:w134:bool)
    n205 = Less?(x=w141, y=w150) -> (x < y?=w149:bool)
    n206 = Less?(x=w152, y=w156) -> (x < y?=w157:bool)
    n207 = Multiply(x=w102, y=5.0) -> (x*y=w429:dbl)
    "N6" <- w429
    n208 = Multiply(x=w103, y=5.0) -> (x*y=w449:dbl)
    "N6-1" <- w449
    n209 = Multiply(x=w93, y=5.0) -> (x*y=w317:dbl)
    "N 14" <- w317
    n210 = Greater?(x=w251, y=w245) -> (0:w246:bool)
    n211 = Less?(x=w126, y=w132) -> (x < y?=w133:bool)
    n212 = Greater?(x=w228, y=w223) -> (0:w224:bool)
    n213 = Greater?(x=w230, y=w235) -> (0:w234:bool)
    n214 = Greater?(x=w253, y=w260) -> (0:w259:bool)
    n215 = Less?(x=w251, y=w248) -> (x < y?=w247:bool)
    n216 = Less?(x=w228, y=w226) -> (x < y?=w225:bool)
    n217 = Multiply(x=w98, y=5.0) -> (x*y=w403:dbl)
    "N12+1" <- w403
    n218 = Less?(x=w230, y=w232) -> (x < y?=w233:bool)
    n219 = Greater?(x=w297, y=w302) -> (0:w303:bool)
    n220 = Less?(x=w253, y=w257) -> (x < y?=w258:bool)
    n221 = Greater?(x=w276, y=w271) -> (0:w272:bool)
    n222 = Greater?(x=w184, y=w189) -> (0:w190:bool)
    n223 = Multiply(x=w99, y=5.0) -> (x*y=w400:dbl)
    "N12" <- w400
    n224 = Add(x=w95, y="Aj7+1") -> (x+y=w340:dbl)
    "B7+1" <- w340
    n225 = Less?(x=w297, y=w305) -> (x < y?=w304:bool)
    n226 = Greater?(x=w277, y=w284) -> (0:w283:bool)
    n227 = Less?(x=w276, y=w274) -> (x < y?=w273:bool)
    n228 = Less?(x=w184, y=w192) -> (x < y?=w191:bool)
    n229 = Greater?(x=w195, y=w200) -> (0:w201:bool)
    n230 = Add(x=w96, y="Aj 7") -> (x+y=w353:dbl)
    "B 7" <- w353
    n231 = Less?(x=w277, y=w281) -> (x < y?=w282:bool)
    n232 = Greater?(x=w380, y=w388) -> (0:w387:bool)
    n233 = Greater?(x=w321, y=w326) -> (0:w327:bool)
    n234 = Less?(x=w195, y=w203) -> (x < y?=w202:bool)
    n235 = Greater?(x=w171, y=w176) -> (0:w177:bool)
    n236 = Add(x=w97, y="Aj 7-1") -> (x+y=w366:dbl)
    "B 7-1" <- w366
    n237 = Greater?(x=w412, y=w419) -> (0:w420:bool)
    n238 = Less?(x=w380, y=w385) -> (x < y?=w386:bool)
    n239 = Less?(x=w321, y=w329) -> (x < y?=w328:bool)
    n240 = Less?(x=w171, y=w179) -> (x < y?=w178:bool)
    n241 = Less?(x=w412, y=w422) -> (x < y?=w421:bool)
    n242 = And(x=w149, y=w148) -> (x .and. y?=w146:bool)
    n243 = Subtract(x=w141, y=w147) -> (x-y=w145:dbl)
    n244 = And(x=w157, y=w158) -> (x .and. y?=w160:bool)
    n245 = Greater?(x=w426, y=w432) -> (0:w431:bool)
    n246 = Subtract(x=w152, y=w159) -> (x-y=w161:dbl)
    n247 = Greater?(x=w445, y=w446) -> (0:w447:bool)
    n248 = Greater?(x=w308, y=w314) -> (0:w315:bool)
    n249 = And(x=w133, y=w134) -> (x .and. y?=w136:bool)
    n250 = Subtract(x=w126, y=w135) -> (x-y=w137:dbl)
    n251 = Less?(x=w426, y=w429) -> (x < y?=w430:bool)
    n252 = Less?(x=w445, y=w449) -> (x < y?=w448:bool)
    n253 = Less?(x=w308, y=w317) -> (x < y?=w316:bool)
    n254 = And(x=w247, y=w246) -> (x .and. y?=w244:bool)
    n255 = Multiply(x=w95, y=5.0) -> (x*y=w343:dbl)
    "N7+1" <- w343
    n256 = Subtract(x=w251, y=w245) -> (x-y=w243:dbl)
    n257 = And(x=w225, y=w224) -> (x .and. y?=w222:bool)
    n258 = Subtract(x=w228, y=w223) -> (x-y=w221:dbl)
    n259 = Greater?(x=w373, y=w406) -> (0:w405:bool)
    n260 = Multiply(x=w96, y=5.0) -> (x*y=w356:dbl)
    "N7" <- w356
    n261 = And(x=w233, y=w234) -> (x .and. y?=w236:bool)
    n262 = And(x=w258, y=w259) -> (x .and. y?=w261:bool)
    n263 = Subtract(x=w230, y=w235) -> (x-y=w237:dbl)
    n264 = Subtract(x=w253, y=w260) -> (x-y=w262:dbl)
    n265 = Greater?(x=w377, y=w397) -> (0:w398:bool)
    n266 = Less?(x=w373, y=w403) -> (x < y?=w404:bool)
    n267 = And(x=w304, y=w303) -> (x .and. y?=w301:bool)
    n268 = Subtract(x=w297, y=w302) -> (x-y=w300:dbl)
    n269 = Multiply(x=w97, y=5.0) -> (x*y=w369:dbl)
    "N7-1" <- w369
    n270 = And(x=w273, y=w272) -> (x .and. y?=w270:bool)
    n271 = Subtract(x=w276, y=w271) -> (x-y=w269:dbl)
    n272 = And(x=w191, y=w190) -> (x .and. y?=w188:bool)
    n273 = Subtract(x=w184, y=w189) -> (x-y=w187:dbl)
    n274 = Less?(x=w377, y=w400) -> (x < y?=w399:bool)
    n275 = And(x=w282, y=w283) -> (x .and. y?=w285:bool)
    n276 = Subtract(x=w277, y=w284) -> (x-y=w286:dbl)
    n277 = And(x=w202, y=w201) -> (x .and. y?=w199:bool)
    n278 = Subtract(x=w195, y=w200) -> (x-y=w198:dbl)
    n279 = And(x=w386, y=w387) -> (x .and. y?=w389:bool)
    n280 = Subtract(x=w380, y=w388) -> (x-y=w390:dbl)
    n281 = And(x=w328, y=w327) -> (x .and. y?=w325:bool)
    n282 = Subtract(x=w321, y=w326) -> (x-y=w324:dbl)
    n283 = And(x=w178, y=w177) -> (x .and. y?=w175:bool)
    n284 = Subtract(x=w171, y=w176) -> (x-y=w174:dbl)
    n285 = Subtract(x=w412, y=w419) -> (x-y=w417:dbl)
    n286 = And(x=w421, y=w420) -> (x .and. y?=w418:bool)
    n287 = And(x=w448, y=w447) -> (x .and. y?=w444:bool)
    n288 = Subtract(x=w426, y=w432) -> (x-y=w434:dbl)
    n289 = And(x=w316, y=w315) -> (x .and. y?=w313:bool)
    n290 = Subtract(x=w445, y=w446) -> (x-y=w443:dbl)
    n291 = Greater?(x=w334, y=w340) -> (0:w341:bool)
    n292 = Subtract(x=w308, y=w314) -> (x-y=w312:dbl)
    n293 = Greater?(x=w345, y=w353) -> (0:w354:bool)
    n294 = And(x=w430, y=w431) -> (x .and. y?=w433:bool)
    n295 = Less?(x=w334, y=w343) -> (x < y?=w342:bool)
    n296 = Less?(x=w345, y=w356) -> (x < y?=w355:bool)
    n297 = Subtract(x=w373, y=w406) -> (x-y=w408:dbl)
    n298 = Greater?(x=w348, y=w366) -> (0:w367:bool)
    n299 = Subtract(x=w377, y=w397) -> (x-y=w395:dbl)
    n300 = And(x=w404, y=w405) -> (x .and. y?=w407:bool)
    n301 = Less?(x=w348, y=w369) -> (x < y?=w368:bool)
    n302 = And(x=w399, y=w398) -> (x .and. y?=w396:bool)
    n303 = And(x=w342, y=w341) -> (x .and. y?=w339:bool)
    n304 = Subtract(x=w334, y=w340) -> (x-y=w338:dbl)
    n305 = And(x=w355, y=w354) -> (x .and. y?=w352:bool)
    n306 = Subtract(x=w345, y=w353) -> (x-y=w351:dbl)
    n307 = And(x=w368, y=w367) -> (x .and. y?=w365:bool)
    n308 = Subtract(x=w348, y=w366) -> (x-y=w364:dbl)
    n309 = case shown="True" w389 {
      tunnel: w390 -> [_ w540]
      tunnel: [0.0 w540] -> w379
      frame False {
      }
      frame True {
      }
    }
    n310 = case shown="True" w418 {
      tunnel: w417 -> [_ w544]
      tunnel: [0.0 w544] -> w411
      frame False {
      }
      frame True {
      }
    }
    n311 = case shown="False" w444 {
      tunnel: w443 -> [_ w552]
      tunnel: [0.0 w552] -> w441
      frame False {
      }
      frame True {
      }
    }
    n312 = case shown="False" w433 {
      tunnel: w434 -> [_ w548]
      tunnel: [0.0 w548] -> w424
      frame False {
      }
      frame True {
      }
    }
    n313 = case shown="True" w407 {
      tunnel: w408 -> [_ w532]
      tunnel: [0.0 w532] -> w371
      frame False {
      }
      frame True {
      }
    }
    n314 = case shown="True" w146 {
      tunnel: w145 -> [_ w464]
      tunnel: [0.0 w464] -> w124
      frame False {
      }
      frame True {
      }
    }
    n315 = case shown="True" w396 {
      tunnel: w395 -> [_ w536]
      tunnel: [0.0 w536] -> w372
      frame False {
      }
      frame True {
      }
    }
    n316 = case shown="True" w160 {
      tunnel: w161 -> [_ w468]
      tunnel: [0.0 w468] -> w125
      frame False {
      }
      frame True {
      }
    }
    n317 = case shown="True" w136 {
      tunnel: w137 -> [_ w460]
      tunnel: [0.0 w460] -> w123
      frame False {
      }
      frame True {
      }
    }
    n318 = case shown="True" w244 {
      tunnel: w243 -> [_ w492]
      tunnel: [0.0 w492] -> w207
      frame False {
      }
      frame True {
      }
    }
    n319 = case shown="True" w222 {
      tunnel: w221 -> [_ w484]
      tunnel: [0.0 w484] -> w205
      frame False {
      }
      frame True {
      }
    }
    n320 = case shown="True" w236 {
      tunnel: w237 -> [_ w488]
      tunnel: [0.0 w488] -> w206
      frame False {
      }
      frame True {
      }
    }
    n321 = case shown="True" w261 {
      tunnel: w262 -> [_ w496]
      tunnel: [0.0 w496] -> w208
      frame False {
      }
      frame True {
      }
    }
    n322 = case shown="True" w301 {
      tunnel: w300 -> [_ w508]
      tunnel: [0.0 w508] -> w292
      frame False {
      }
      frame True {
      }
    }
    n323 = case shown="True" w270 {
      tunnel: w269 -> [_ w500]
      tunnel: [0.0 w500] -> w209
      frame False {
      }
      frame True {
      }
    }
    n324 = case shown="True" w313 {
      tunnel: w312 -> [_ w512]
      tunnel: [0.0 w512] -> w293
      frame False {
      }
      frame True {
      }
    }
    n325 = case shown="True" w188 {
      tunnel: w187 -> [_ w476]
      tunnel: [0.0 w476] -> w167
      frame False {
      }
      frame True {
      }
    }
    n326 = case shown="True" w285 {
      tunnel: w286 -> [_ w504]
      tunnel: [0.0 w504] -> w210
      frame False {
      }
      frame True {
      }
    }
    n327 = case shown="True" w325 {
      tunnel: w324 -> [_ w516]
      tunnel: [0.0 w516] -> w294
      frame False {
      }
      frame True {
      }
    }
    n328 = case shown="True" w339 {
      tunnel: w338 -> [_ w520]
      tunnel: [0.0 w520] -> w331
      frame False {
      }
      frame True {
      }
    }
    n329 = case shown="True" w199 {
      tunnel: w198 -> [_ w480]
      tunnel: [0.0 w480] -> w168
      frame False {
      }
      frame True {
      }
    }
    n330 = case shown="True" w352 {
      tunnel: w351 -> [_ w524]
      tunnel: [0.0 w524] -> w332
      frame False {
      }
      frame True {
      }
    }
    n331 = case shown="True" w175 {
      tunnel: w174 -> [_ w472]
      tunnel: [0.0 w472] -> w166
      frame False {
      }
      frame True {
      }
    }
    n332 = case shown="False" w365 {
      tunnel: w364 -> [_ w528]
      tunnel: [0.0 w528] -> w358
      frame False {
      }
      frame True {
      }
    }
    n333 = Build Array(w358, w332, w331, w294, w293, w292) -> (w359:dbl[])
    "7 Hz" <- w359
    n334 = Build Array(w441, w424, w411, w379, w372, w371) -> (w439:dbl[])
    "6 Hz" <- w439
    n335 = Array Max & Min(array=w359) -> (max value=w122:dbl, max index (indices)=→"Max Index 7":i32)  [unwired: 2 out]
    "PSD max 7" <- w122
    n336 = Array Max & Min(array=w439) -> (max value=w119:dbl, max index (indices)=→"Max Index 6":i32)  [unwired: 2 out]
    "PSD max 6" <- w119
    n337 = Build Array(w210, w209, w208, w207, w206, w205) -> (w211:dbl[])
    "8 Hz" <- w211
    n338 = Build Array(w168, w167, w166, w125, w124, w123) -> (w169:dbl[])
    "9 Hz" <- w169
    n339 = Array Max & Min(array=w211) -> (max value=w121:dbl, max index (indices)=→"Max Index 8":i32)  [unwired: 2 out]
    "PSD max 8" <- w121
    n340 = Array Max & Min(array=w169) -> (max value=w120:dbl, max index (indices)=→"Max Index 9":i32)  [unwired: 2 out]
    "PSD max 9" <- w120
    n341 = Build Array(w119, w122, w121, w120) -> (w118:dbl[])
    n342 = Array Max & Min(array=w118) -> (max value=w116:dbl, max index (indices)=w117:i32)  [unwired: 2 out]
    "max value" <- w116
    "PSD MAX" <- w116
    n343 = Greater?(x=w116, y=0.0 ("x")) -> (0:w114:bool)
    n344 = case shown="True" w114 {
      tunnel: w117 -> [_ w458]
      tunnel: [555 w458] -> w106
      frame False {
      }
      frame True {
      }
    }
    "Index ที่มากที่สุด" <- w106
    n345 = Equal?(x=0, y=w106) -> (x = y?=→"6 HZ 2" →"Emotion 4" →"Emotion 8" →"Emotion 16":bool)
    n346 = Equal?(x=1, y=w106) -> (x = y?=→"7 HZ" →"Emotion 5" →"Emotion 9" →"Emotion 17":bool)
    n347 = Equal?(x=2, y=w106) -> (x = y?=→"8 HZ" →"Emotion 6" →"Emotion 10" →"Emotion 19":bool)
    n348 = Equal?(x=3, y=w106) -> (x = y?=→"9 HZ" →"Emotion 7" →"Emotion 11" →"Emotion 18":bool)
    n349 = Equal?(x=555, y=w106) -> (x = y?=→"555":bool)
  }
  n350 = while {
    stop <- FALSE stop-if-true
    n351 = event shown="[4] \"Emer\": Value Change" {
      selector: _ -> [_ _ _ _ _ _ _]
      dyn-events: _ -> [_ _ _ _ _ _ _]
      timeout: _ -> [_ _ _ _ _ _ _]
      event Timeout {
        n352 = event-data() -> ()  [unwired: 1 in, 3 out]
      }
      event Value Change {
        n353 = event-data() -> ()  [unwired: 1 in, 6 out]
        n354 = local write "Tab Control"(enum32{"TAB 1", "TAB 2", "TAB 3", "TAB 4"}."TAB 2" ("Tab Control")) -> ()
      }
      event Value Change {
        n355 = event-data() -> ()  [unwired: 1 in, 6 out]
        n356 = local write "Tab Control"(enum32{"TAB 1", "TAB 2", "TAB 3", "TAB 4"}."TAB 3" ("Tab Control")) -> ()
      }
      event Value Change {
        n357 = event-data() -> ()  [unwired: 1 in, 6 out]
        n358 = local write "Tab Control"(T2."TAB 1" ("Tab Control")) -> ()
      }
      event "Emer": Value Change {
        n359 = event-data() -> ()  [unwired: 1 in, 6 out]
        n360 = local write "Tab Control"(enum32{"TAB 1", "TAB 2", "TAB 3", "TAB 4"}."TAB 4" ("Tab Control")) -> ()
      }
      event Value Change {
        n361 = event-data() -> ()  [unwired: 1 in, 6 out]
        n362 = local write "Tab Control"(enum32{"TAB 1", "TAB 2", "TAB 3", "TAB 4"}."TAB 4" ("Tab Control")) -> ()
      }
      event "BACK_Page4": Value Change {
        n363 = event-data() -> ()  [unwired: 1 in, 6 out]
        n364 = local write "Tab Control"(enum32{"TAB 1", "TAB 2", "TAB 3", "TAB 4"}."TAB 1" ("Tab Control")) -> ()
      }
    }
  }
  n365 = call <vilib>:"Read JPEG File.vi"("path to JPEG file"="Activity 1") -> ("image data"=w13:T1)  [unwired: 8 in, 2 out]
  "image data" <- w13
  n366 = call <vilib>:"Read JPEG File.vi"("path to JPEG file"="Activity 3") -> ("image data"=w7:T1)  [unwired: 8 in, 2 out]
  n367 = call <vilib>:"Read JPEG File.vi"("path to JPEG file"="Activity 2") -> ("image data"=w12:T1)  [unwired: 8 in, 2 out]
  n368 = call <vilib>:"Draw Flattened Pixmap.vi"("image data"=w13) -> ("new picture"=→"new picture":picture)  [unwired: 8 in]
  n369 = call <vilib>:"Draw Flattened Pixmap.vi"("image data"=w7) -> ("new picture"=→"new picture 3":picture)  [unwired: 8 in]
  n370 = call <vilib>:"Draw Flattened Pixmap.vi"("image data"=w12) -> ("new picture"=→"new picture 2":picture)  [unwired: 8 in]
  n371 = local read "Tab Control"() -> (w2:T2)
  n372 = Obtain Notifier(notification data type=w2) -> (notifier out=w1:refnum<notifier>, error out=w4:errorcluster)  [unwired: 3 in, 1 out]
  n373 = while {
    tunnel: w1 -> [w572]
    stop <- FALSE stop-if-true
    n374 = Wait on Notification(notifier=w572) -> (notification=w571:T2)  [unwired: 3 in, 3 out]
    n375 = case shown="\"TAB 4\"" w571 {
      frame "TAB 1" {
        n376 = while {
          stop <- w623 stop-if-true
          n377 = local read "Baseline"() -> (w615:bool)
          n378 = feedback #25() -> (w635:i32)  [unwired: 1 in]
          n379 = case shown="True" w615 {
            tunnel: [w659 w660] -> w636
            tunnel: w635 -> [w659 w661]
            frame False {
            }
            frame True {
              n380 = Increment(x=w661) -> (x+1=w660:i32)
            }
          }
          n381 = case shown="0, Default" w636 {
            selector: w636 -> [w638 w642 w643 w650 w654 w657]
            tunnel: [w638 w642 w643 w650 w654 w656] -> w634
            frame 0, Default {
              w637 = FALSE ("B")
              n382 = local write "ele"(w637) -> ()
              n383 = local write "call"(w637) -> ()
              n384 = local write "commu"(w637) -> ()
              n385 = local write "Emotion"(w637) -> ()
              n386 = local write "Activity"(w637) -> ()
              n387 = local write "ACC"(w637) -> ()
            }
            frame 1 {
              n388 = local write "Emer"(FALSE) -> ()
              n389 = Wait (ms)(milliseconds to wait=u32 1500 ("millisecond timer value")) -> ()  [unwired: 1 out]
              "ele" <- TRUE
            }
            frame 2 {
              n390 = local write "ele"(FALSE) -> ()
              n391 = Wait (ms)(milliseconds to wait=u32 1000) -> ()  [unwired: 1 out]
              "call" <- TRUE
            }
            frame 3 {
              n392 = local write "call"(FALSE) -> ()
              n393 = Wait (ms)(milliseconds to wait=u32 1000) -> ()  [unwired: 1 out]
              "commu" <- TRUE
            }
            frame 4 {
              n394 = local write "commu"(FALSE) -> ()
              n395 = Wait (ms)(milliseconds to wait=u32 1000) -> ()  [unwired: 1 out]
              "Emer" <- TRUE
            }
            frame 5 {
              n396 = Subtract(x=w657, y=5 ("x")) -> (x-y=w656:i32)
              n397 = Wait (ms)(milliseconds to wait=u32 1200 ("millisecond timer value")) -> ()  [unwired: 1 out]
            }
          }
          n398 = feedback-in #25(w634) -> ()
          n399 = local read "Tab Control"() -> (w625:T2)
          n400 = Equal?(x=w625, y=T2."TAB 2" ("Tab Control")) -> (x = y?=w633:bool)
          n401 = Equal?(x=w625, y=T2."TAB 6" ("Tab Control")) -> (x = y?=w627:bool)
          n402 = Equal?(x=w625, y=T2."TAB 3" ("Tab Control")) -> (x = y?=w632:bool)
          n403 = Equal?(x=w625, y=T2."TAB 4" ("Tab Control")) -> (x = y?=w631:bool)
          n404 = Equal?(x=w625, y=T2."TAB 7" ("Tab Control")) -> (x = y?=w626:bool)
          n405 = Equal?(x=w625, y=T2."TAB 5" ("Tab Control")) -> (x = y?=w630:bool)
          n406 = Or(x=w633, y=w632) -> (x .or. y?=w629:bool)
          n407 = Or(x=w627, y=w626) -> (x .or. y?=w622:bool)
          n408 = Or(x=w631, y=w630) -> (x .or. y?=w628:bool)
          n409 = Or(x=w629, y=w628) -> (x .or. y?=w624:bool)
          n410 = Or(x=w624, y=w622) -> (x .or. y?=w623:bool)
        }
        n411 = while {
          stop <- w593 stop-if-true
          n412 = flat-sequence {
            frame #0 {
              n413 = while {
                stop <- w596 stop-if-true
                n414 = local read "Clear1"() -> (w594:bool)
                n415 = local read "ele"() -> (w595:T3)
                n416 = Or(x=w595, y=w594) -> (x .or. y?=w596:T3)
              }
            }
            frame #1 {
              n417 = while {
                stop <- w602 stop-if-true
                n418 = local read "Index ที่มากที่สุด"() -> (w601:i32)
                n419 = local read "Clear1"() -> (w597:bool)
                n420 = local read "call"() -> (w599:T4)
                n421 = Equal?(x=w601, y=0) -> (x = y?=→"ele":bool)
                n422 = Or(x=w599, y=w597) -> (x .or. y?=w602:T4)
              }
            }
            frame #2 {
              n423 = while {
                stop <- w605 stop-if-true
                n424 = local read "Index ที่มากที่สุด"() -> (w608:i32)
                n425 = local read "commu"() -> (w603:T5)
                n426 = local read "Clear1"() -> (w604:bool)
                n427 = Equal?(x=w608, y=1) -> (x = y?=→"call":bool)
                n428 = Or(x=w603, y=w604) -> (x .or. y?=w605:T5)
              }
            }
            frame #3 {
              n429 = while {
                stop <- w609 stop-if-true
                n430 = local read "Index ที่มากที่สุด"() -> (w614:i32)
                n431 = local read "Clear1"() -> (w610:bool)
                n432 = local read "Emer"() -> (w611:bool)
                n433 = Equal?(x=w614, y=2) -> (x = y?=→"com":bool)
                n434 = Or(x=w611, y=w610) -> (x .or. y?=w609:bool)
              }
            }
          }
          n435 = local read "Clear1"() -> (w593:bool)
        }
        n436 = while {
          stop <- w574 stop-if-true
          n437 = local read "Tab Control"() -> (w584:T2)
          n438 = Equal?(x=w584, y=T2."TAB 2" ("Tab Control")) -> (x = y?=w592:bool)
          n439 = Equal?(x=w584, y=T2."TAB 3" ("Tab Control")) -> (x = y?=w591:bool)
          n440 = Equal?(x=w584, y=T2."TAB 4" ("Tab Control")) -> (x = y?=w590:bool)
          n441 = Equal?(x=w584, y=T2."TAB 5" ("Tab Control")) -> (x = y?=w580:bool)
          n442 = Equal?(x=w584, y=T2."TAB 6" ("Tab Control")) -> (x = y?=w579:bool)
          n443 = Equal?(x=w584, y=T2."TAB 7" ("Tab Control")) -> (x = y?=w576:bool)
          n444 = Or(x=w592, y=w591) -> (x .or. y?=w589:bool)
          n445 = Or(x=w591, y=w590) -> (x .or. y?=w588:bool)
          n446 = Or(x=w580, y=w579) -> (x .or. y?=w577:bool)
          n447 = Or(x=w589, y=w588) -> (x .or. y?=w578:bool)
          n448 = Or(x=w577, y=w576) -> (x .or. y?=w575:bool)
          n449 = Or(x=w578, y=w575) -> (x .or. y?=w574:bool)
          "Clear1" <- w574
        }
      }
      frame "TAB 2" {
        n450 = while {
          stop <- w717 stop-if-true
          n451 = local read "Baseline"() -> (w709:bool)
          n452 = feedback #26() -> (w729:i32)  [unwired: 1 in]
          n453 = case shown="True" w709 {
            tunnel: [w753 w754] -> w730
            tunnel: w729 -> [w753 w755]
            frame False {
            }
            frame True {
              n454 = Increment(x=w755) -> (x+1=w754:i32)
            }
          }
          n455 = case shown="1" w730 {
            selector: w730 -> [w732 w736 w739 w744 w748 w751]
            tunnel: [w732 w736 w739 w744 w748 w750] -> w728
            frame 0, Default {
              w731 = FALSE ("B")
              n456 = local write "cummu_back"(w731) -> ()
              n457 = local write "cummu_2"(w731) -> ()
              n458 = local write "cummu_1"(w731) -> ()
              n459 = local write "8-2"(w731) -> ()
            }
            frame 1 {
              n460 = local write "cummu_back"(FALSE) -> ()
              n461 = Wait (ms)(milliseconds to wait=u32 1500 ("millisecond timer value")) -> ()  [unwired: 1 out]
              "cummu_1" <- TRUE
            }
            frame 2 {
              n462 = local write "cummu_1"(FALSE) -> ()
              n463 = Wait (ms)(milliseconds to wait=u32 1000) -> ()  [unwired: 1 out]
              "cummu_2" <- TRUE
            }
            frame 3 {
              n464 = local write "cummu_2"(FALSE) -> ()
              n465 = Wait (ms)(milliseconds to wait=u32 1000) -> ()  [unwired: 1 out]
              "8-2" <- TRUE
            }
            frame 4 {
              n466 = local write "8-2"(FALSE) -> ()
              n467 = Wait (ms)(milliseconds to wait=u32 1000) -> ()  [unwired: 1 out]
              "cummu_back" <- TRUE
            }
            frame 5 {
              n468 = Subtract(x=w751, y=5 ("x")) -> (x-y=w750:i32)
              n469 = Wait (ms)(milliseconds to wait=u32 1200 ("millisecond timer value")) -> ()  [unwired: 1 out]
            }
          }
          n470 = feedback-in #26(w728) -> ()
          n471 = local read "Tab Control"() -> (w719:T2)
          n472 = Equal?(x=w719, y=T2."TAB 1" ("Tab Control")) -> (x = y?=w727:bool)
          n473 = Equal?(x=w719, y=T2."TAB 6" ("Tab Control")) -> (x = y?=w721:bool)
          n474 = Equal?(x=w719, y=T2."TAB 3" ("Tab Control")) -> (x = y?=w726:bool)
          n475 = Equal?(x=w719, y=T2."TAB 4" ("Tab Control")) -> (x = y?=w725:bool)
          n476 = Equal?(x=w719, y=T2."TAB 7" ("Tab Control")) -> (x = y?=w720:bool)
          n477 = Equal?(x=w719, y=T2."TAB 5" ("Tab Control")) -> (x = y?=w724:bool)
          n478 = Or(x=w727, y=w726) -> (x .or. y?=w723:bool)
          n479 = Or(x=w721, y=w720) -> (x .or. y?=w716:bool)
          n480 = Or(x=w725, y=w724) -> (x .or. y?=w722:bool)
          n481 = Or(x=w723, y=w722) -> (x .or. y?=w718:bool)
          n482 = Or(x=w718, y=w716) -> (x .or. y?=w717:bool)
        }
        n483 = while {
          stop <- w681 stop-if-true
          n484 = flat-sequence {
            frame #0 {
              n485 = while {
                stop <- w684 stop-if-true
                n486 = local read "cummu_1"() -> (w682:bool)
                n487 = local read "Clear2"() -> (w683:bool)
                n488 = Or(x=w682, y=w683) -> (x .or. y?=w684:bool)
              }
            }
            frame #1 {
              n489 = while {
                stop <- w690 stop-if-true
                n490 = local read "Index ที่มากที่สุด"() -> (w689:i32)
                n491 = local read "cummu_2"() -> (w685:bool)
                n492 = local read "Clear2"() -> (w687:bool)
                n493 = Equal?(x=w689, y=0) -> (x = y?=→"Activity":bool)
                n494 = Or(x=w685, y=w687) -> (x .or. y?=w690:bool)
              }
            }
            frame #2 {
              n495 = while {
                stop <- w694 stop-if-true
                n496 = local read "Index ที่มากที่สุด"() -> (w696:i32)
                n497 = local read "Clear2"() -> (w693:bool)
                n498 = local read "8-2"() -> (w691:bool)
                n499 = Equal?(x=w696, y=1) -> (x = y?=→"Emotion":bool)
                n500 = Or(x=w691, y=w693) -> (x .or. y?=w694:bool)
              }
            }
            frame #3 {
              n501 = while {
                stop <- w699 stop-if-true
                n502 = local read "Index ที่มากที่สุด"() -> (w702:i32)
                n503 = local read "cummu_back"() -> (w697:bool)
                n504 = local read "Clear2"() -> (w700:bool)
                n505 = Equal?(x=w702, y=2) -> (x = y?=→"ACC":bool)
                n506 = Or(x=w697, y=w700) -> (x .or. y?=w699:bool)
              }
            }
            frame #4 {
              n507 = while {
                stop <- FALSE stop-if-true
                n508 = local read "Index ที่มากที่สุด"() -> (w708:i32)
                n509 = local read "cummu_1"() -> (w704:bool)
                n510 = local read "Clear2"() -> (w705:bool)
                n511 = Equal?(x=w708, y=3) -> (x = y?=→"back_page2":bool)
                n512 = Or(x=w704, y=w705) -> ()  [unwired: 1 out]
              }
            }
          }
          n513 = local read "Clear2"() -> (w681:bool)
        }
        n514 = while {
          stop <- w662 stop-if-true
          n515 = local read "Tab Control"() -> (w672:T2)
          n516 = Equal?(x=w672, y=T2."TAB 1" ("Tab Control")) -> (x = y?=w680:bool)
          n517 = Equal?(x=w672, y=T2."TAB 3" ("Tab Control")) -> (x = y?=w679:bool)
          n518 = Equal?(x=w672, y=T2."TAB 4" ("Tab Control")) -> (x = y?=w678:bool)
          n519 = Equal?(x=w672, y=T2."TAB 5" ("Tab Control")) -> (x = y?=w668:bool)
          n520 = Equal?(x=w672, y=T2."TAB 6" ("Tab Control")) -> (x = y?=w667:bool)
          n521 = Equal?(x=w672, y=T2."TAB 7" ("Tab Control")) -> (x = y?=w664:bool)
          n522 = Or(x=w680, y=w679) -> (x .or. y?=w677:bool)
          n523 = Or(x=w679, y=w678) -> (x .or. y?=w676:bool)
          n524 = Or(x=w668, y=w667) -> (x .or. y?=w665:bool)
          n525 = Or(x=w677, y=w676) -> (x .or. y?=w666:bool)
          n526 = Or(x=w665, y=w664) -> (x .or. y?=w663:bool)
          n527 = Or(x=w666, y=w663) -> (x .or. y?=w662:bool)
          "Clear2" <- w662
        }
      }
      frame "TAB 3" {
        n528 = while {
          stop <- w811 stop-if-true
          n529 = local read "Baseline"() -> (w803:bool)
          n530 = feedback #27() -> (w823:i32)  [unwired: 1 in]
          n531 = case shown="True" w803 {
            tunnel: [w847 w848] -> w824
            tunnel: w823 -> [w847 w849]
            frame False {
            }
            frame True {
              n532 = Increment(x=w849) -> (x+1=w848:i32)
            }
          }
          n533 = case shown="1" w824 {
            selector: w824 -> [w826 w830 w833 w838 w842 w845]
            tunnel: [w826 w830 w833 w838 w842 w844] -> w822
            frame 0, Default {
              w825 = FALSE ("B")
              n534 = local write "call_back"(w825) -> ()
              n535 = local write "call_1"(w825) -> ()
              n536 = local write "call_2"(w825) -> ()
              n537 = local write "call_3"(w825) -> ()
            }
            frame 1 {
              n538 = local write "call_back"(FALSE) -> ()
              n539 = Wait (ms)(milliseconds to wait=u32 1500 ("millisecond timer value")) -> ()  [unwired: 1 out]
              "call_1" <- TRUE
            }
            frame 2 {
              n540 = local write "call_1"(FALSE) -> ()
              n541 = Wait (ms)(milliseconds to wait=u32 1000) -> ()  [unwired: 1 out]
              "call_2" <- TRUE
            }
            frame 3 {
              n542 = local write "call_2"(FALSE) -> ()
              n543 = Wait (ms)(milliseconds to wait=u32 1000) -> ()  [unwired: 1 out]
              "call_3" <- TRUE
            }
            frame 4 {
              n544 = local write "call_3"(FALSE) -> ()
              n545 = Wait (ms)(milliseconds to wait=u32 1000) -> ()  [unwired: 1 out]
              "call_back" <- TRUE
            }
            frame 5 {
              n546 = Subtract(x=w845, y=5 ("x")) -> (x-y=w844:i32)
              n547 = Wait (ms)(milliseconds to wait=u32 1200 ("millisecond timer value")) -> ()  [unwired: 1 out]
            }
          }
          n548 = feedback-in #27(w822) -> ()
          n549 = local read "Tab Control"() -> (w813:T2)
          n550 = Equal?(x=w813, y=T2."TAB 1" ("Tab Control")) -> (x = y?=w821:bool)
          n551 = Equal?(x=w813, y=T2."TAB 6" ("Tab Control")) -> (x = y?=w815:bool)
          n552 = Equal?(x=w813, y=T2."TAB 2" ("Tab Control")) -> (x = y?=w820:bool)
          n553 = Equal?(x=w813, y=T2."TAB 4" ("Tab Control")) -> (x = y?=w819:bool)
          n554 = Equal?(x=w813, y=T2."TAB 7" ("Tab Control")) -> (x = y?=w814:bool)
          n555 = Equal?(x=w813, y=T2."TAB 5" ("Tab Control")) -> (x = y?=w818:bool)
          n556 = Or(x=w821, y=w820) -> (x .or. y?=w817:bool)
          n557 = Or(x=w815, y=w814) -> (x .or. y?=w810:bool)
          n558 = Or(x=w819, y=w818) -> (x .or. y?=w816:bool)
          n559 = Or(x=w817, y=w816) -> (x .or. y?=w812:bool)
          n560 = Or(x=w812, y=w810) -> (x .or. y?=w811:bool)
        }
        n561 = while {
          stop <- w775 stop-if-true
          n562 = flat-sequence {
            frame #0 {
              n563 = while {
                stop <- w778 stop-if-true
                n564 = local read "Clear 3"() -> (w777:bool)
                n565 = local read "call_1"() -> (w776:bool)
                n566 = Or(x=w776, y=w777) -> (x .or. y?=w778:bool)
              }
            }
            frame #1 {
              n567 = while {
                stop <- w784 stop-if-true
                n568 = local read "Index ที่มากที่สุด"() -> (w783:i32)
                n569 = local read "Clear 3"() -> (w779:bool)
                n570 = local read "call_2"() -> (w780:bool)
                n571 = Equal?(x=w783, y=0) -> (x = y?=→"1":bool)
                n572 = Or(x=w780, y=w779) -> (x .or. y?=w784:bool)
              }
            }
            frame #2 {
              n573 = while {
                stop <- w785 stop-if-true
                n574 = local read "Index ที่มากที่สุด"() -> (w790:i32)
                n575 = local read "Clear 3"() -> (w787:bool)
                n576 = local read "call_3"() -> (w786:bool)
                n577 = Equal?(x=w790, y=1) -> (x = y?=→"1 2":bool)
                n578 = Or(x=w786, y=w787) -> (x .or. y?=w785:bool)
              }
            }
            frame #3 {
              n579 = while {
                stop <- w794 stop-if-true
                n580 = local read "Index ที่มากที่สุด"() -> (w796:i32)
                n581 = local read "call_back"() -> (w791:bool)
                n582 = local read "Clear 3"() -> (w792:bool)
                n583 = Equal?(x=w796, y=2) -> (x = y?=→"1 3":bool)
                n584 = Or(x=w791, y=w792) -> (x .or. y?=w794:bool)
              }
            }
            frame #4 {
              n585 = while {
                stop <- FALSE stop-if-true
                n586 = local read "Index ที่มากที่สุด"() -> (w802:i32)
                n587 = local read "call_1"() -> (w797:bool)
                n588 = local read "Clear 3"() -> (w798:bool)
                n589 = Equal?(x=w802, y=3) -> (x = y?=→"call_back":bool)
                n590 = Or(x=w797, y=w798) -> ()  [unwired: 1 out]
              }
            }
          }
          n591 = local read "Clear 3"() -> (w775:bool)
        }
        n592 = while {
          stop <- w756 stop-if-true
          n593 = local read "Tab Control"() -> (w766:T2)
          n594 = Equal?(x=w766, y=T2."TAB 1" ("Tab Control")) -> (x = y?=w774:bool)
          n595 = Equal?(x=w766, y=T2."TAB 2" ("Tab Control")) -> (x = y?=w773:bool)
          n596 = Equal?(x=w766, y=T2."TAB 4" ("Tab Control")) -> (x = y?=w772:bool)
          n597 = Equal?(x=w766, y=T2."TAB 5" ("Tab Control")) -> (x = y?=w762:bool)
          n598 = Equal?(x=w766, y=T2."TAB 6" ("Tab Control")) -> (x = y?=w761:bool)
          n599 = Equal?(x=w766, y=T2."TAB 7" ("Tab Control")) -> (x = y?=w758:bool)
          n600 = Or(x=w774, y=w773) -> (x .or. y?=w771:bool)
          n601 = Or(x=w773, y=w772) -> (x .or. y?=w770:bool)
          n602 = Or(x=w762, y=w761) -> (x .or. y?=w759:bool)
          n603 = Or(x=w771, y=w770) -> (x .or. y?=w760:bool)
          n604 = Or(x=w759, y=w758) -> (x .or. y?=w757:bool)
          n605 = Or(x=w760, y=w757) -> (x .or. y?=w756:bool)
          "Clear 3" <- w756
        }
      }
      frame "TAB 4" {
        n606 = while {
          stop <- w905 stop-if-true
          n607 = local read "Baseline"() -> (w897:bool)
          n608 = feedback #28() -> (w917:i32)  [unwired: 1 in]
          n609 = case shown="True" w897 {
            tunnel: [w941 w942] -> w918
            tunnel: w917 -> [w941 w943]
            frame False {
            }
            frame True {
              n610 = Increment(x=w943) -> (x+1=w942:i32)
            }
          }
          n611 = case shown="1" w918 {
            selector: w918 -> [w920 w924 w927 w932 w936 w939]
            tunnel: [w920 w924 w927 w932 w936 w938] -> w916
            frame 0, Default {
              w919 = FALSE ("B")
              n612 = local write "ele_back"(w919) -> ()
              n613 = local write "ele_1"(w919) -> ()
              n614 = local write "ele_2"(w919) -> ()
              n615 = local write "ele_3"(w919) -> ()
            }
            frame 1 {
              n616 = local write "ele_back"(FALSE) -> ()
              n617 = Wait (ms)(milliseconds to wait=u32 1500 ("millisecond timer value")) -> ()  [unwired: 1 out]
              "ele_1" <- TRUE
            }
            frame 2 {
              n618 = local write "ele_1"(FALSE) -> ()
              n619 = Wait (ms)(milliseconds to wait=u32 1000) -> ()  [unwired: 1 out]
              "ele_2" <- TRUE
            }
            frame 3 {
              n620 = local write "ele_2"(FALSE) -> ()
              n621 = Wait (ms)(milliseconds to wait=u32 1000) -> ()  [unwired: 1 out]
              "ele_3" <- TRUE
            }
            frame 4 {
              n622 = local write "ele_3"(FALSE) -> ()
              n623 = Wait (ms)(milliseconds to wait=u32 1000) -> ()  [unwired: 1 out]
              "ele_back" <- TRUE
            }
            frame 5 {
              n624 = Subtract(x=w939, y=5 ("x")) -> (x-y=w938:i32)
              n625 = Wait (ms)(milliseconds to wait=u32 1200 ("millisecond timer value")) -> ()  [unwired: 1 out]
            }
          }
          n626 = feedback-in #28(w916) -> ()
          n627 = local read "Tab Control"() -> (w907:T2)
          n628 = Equal?(x=w907, y=T2."TAB 1" ("Tab Control")) -> (x = y?=w915:bool)
          n629 = Equal?(x=w907, y=T2."TAB 6" ("Tab Control")) -> (x = y?=w909:bool)
          n630 = Equal?(x=w907, y=T2."TAB 2" ("Tab Control")) -> (x = y?=w914:bool)
          n631 = Equal?(x=w907, y=T2."TAB 3" ("Tab Control")) -> (x = y?=w913:bool)
          n632 = Equal?(x=w907, y=T2."TAB 7" ("Tab Control")) -> (x = y?=w908:bool)
          n633 = Equal?(x=w907, y=T2."TAB 5" ("Tab Control")) -> (x = y?=w912:bool)
          n634 = Or(x=w915, y=w914) -> (x .or. y?=w911:bool)
          n635 = Or(x=w909, y=w908) -> (x .or. y?=w904:bool)
          n636 = Or(x=w913, y=w912) -> (x .or. y?=w910:bool)
          n637 = Or(x=w911, y=w910) -> (x .or. y?=w906:bool)
          n638 = Or(x=w906, y=w904) -> (x .or. y?=w905:bool)
        }
        n639 = while {
          stop <- w869 stop-if-true
          n640 = flat-sequence {
            frame #0 {
              n641 = while {
                stop <- w872 stop-if-true
                n642 = local read "Clear4"() -> (w871:bool)
                n643 = local read "ele_1"() -> (w870:bool)
                n644 = Or(x=w870, y=w871) -> (x .or. y?=w872:bool)
              }
            }
            frame #1 {
              n645 = while {
                stop <- w878 stop-if-true
                n646 = local read "Index ที่มากที่สุด"() -> (w877:i32)
                n647 = local read "Clear4"() -> (w875:bool)
                n648 = local read "ele_2"() -> (w873:bool)
                n649 = Equal?(x=w877, y=0) -> (x = y?=→"ele_1":bool)
                n650 = Or(x=w873, y=w875) -> (x .or. y?=w878:bool)
              }
            }
            frame #2 {
              n651 = while {
                stop <- w881 stop-if-true
                n652 = local read "Index ที่มากที่สุด"() -> (w884:i32)
                n653 = local read "Clear4"() -> (w882:bool)
                n654 = local read "ele_3"() -> (w879:bool)
                n655 = Equal?(x=w884, y=1) -> (x = y?=→"ele_2":bool)
                n656 = Or(x=w879, y=w882) -> (x .or. y?=w881:bool)
              }
            }
            frame #3 {
              n657 = while {
                stop <- w888 stop-if-true
                n658 = local read "Index ที่มากที่สุด"() -> (w890:i32)
                n659 = local read "ele_back"() -> (w885:bool)
                n660 = local read "Clear4"() -> (w887:bool)
                n661 = Equal?(x=w890, y=2) -> (x = y?=→"ele_3":bool)
                n662 = Or(x=w885, y=w887) -> (x .or. y?=w888:bool)
              }
            }
            frame #4 {
              n663 = while {
                stop <- FALSE stop-if-true
                n664 = local read "Index ที่มากที่สุด"() -> (w896:i32)
                n665 = local read "Clear4"() -> (w893:bool)
                n666 = local read "ele_1"() -> (w891:bool)
                n667 = Equal?(x=w896, y=3) -> (x = y?=→"BACK_Page4":bool)
                n668 = Or(x=w891, y=w893) -> ()  [unwired: 1 out]
              }
            }
          }
          n669 = local read "Clear4"() -> (w869:bool)
        }
        n670 = while {
          stop <- w850 stop-if-true
          n671 = local read "Tab Control"() -> (w860:T2)
          n672 = Equal?(x=w860, y=T2."TAB 1" ("Tab Control")) -> (x = y?=w868:bool)
          n673 = Equal?(x=w860, y=T2."TAB 2" ("Tab Control")) -> (x = y?=w867:bool)
          n674 = Equal?(x=w860, y=T2."TAB 3" ("Tab Control")) -> (x = y?=w866:bool)
          n675 = Equal?(x=w860, y=T2."TAB 5" ("Tab Control")) -> (x = y?=w856:bool)
          n676 = Equal?(x=w860, y=T2."TAB 6" ("Tab Control")) -> (x = y?=w855:bool)
          n677 = Equal?(x=w860, y=T2."TAB 7" ("Tab Control")) -> (x = y?=w852:bool)
          n678 = Or(x=w868, y=w867) -> (x .or. y?=w865:bool)
          n679 = Or(x=w867, y=w866) -> (x .or. y?=w864:bool)
          n680 = Or(x=w856, y=w855) -> (x .or. y?=w853:bool)
          n681 = Or(x=w865, y=w864) -> (x .or. y?=w854:bool)
          n682 = Or(x=w853, y=w852) -> (x .or. y?=w851:bool)
          n683 = Or(x=w854, y=w851) -> (x .or. y?=w850:bool)
          "Clear4" <- w850
        }
      }
    }
  }
  n684 = while {
    tunnel: w1 -> [w948]
    tunnel: [w947] -> w5
    tunnel: w4 -> [w946]
    tunnel: [w945] -> w3
    stop <- FALSE stop-if-true
    n685 = case shown="\"TAB 7\"" "Tab Control" {
      selector: "Tab Control" -> [w952 w976 w985 w994 w1006 w1016 w1026]
      tunnel: [w951 w973 w982 w992 w1002 w1012 w1022] -> w944
      frame "TAB 1", Default {
        n686 = local read "Index ที่มากที่สุด"() -> (w953:i32)
        n687 = local read "commu"() -> (w954:T5)
        n688 = Add(x=w952, y=3) -> (x+y=w971:u32)
        n689 = local read "Index ที่มากที่สุด"() -> (w959:i32)
        n690 = local read "ele"() -> (w958:T3)
        n691 = local read "Index ที่มากที่สุด"() -> (w957:i32)
        n692 = Equal?(x=w953, y=2) -> (x = y?=w969:bool)
        n693 = Increment(x=w952) -> (x+1=w963:T2)
        n694 = local read "call"() -> (w956:T4)
        n695 = And(x=w954, y=w969) -> (x .and. y?=w970:T5)
        n696 = Equal?(x=w959, y=0) -> (x = y?=w967:bool)
        n697 = Equal?(x=w957, y=1) -> (x = y?=w968:bool)
        n698 = And(x=w956, y=w968) -> (x .and. y?=w964:T4)
        n699 = And(x=w958, y=w967) -> (x .and. y?=w965:T3)
        n700 = Select(t=w971, s=w970, f=w952) -> (s? t:f=w972:u32)
        n701 = Select(t=w971, s=w964, f=w972) -> (s? t:f=w966:u32)
        n702 = Select(t=w963, s=w965, f=w966) -> (s? t:f=w951:u32)
      }
      frame "TAB 2" {
        n703 = local read "Index ที่มากที่สุด"() -> (w979:i32)
        n704 = local read "back_page2"() -> (w980:T7)
        n705 = Decrement(x=w976) -> (x-1=w978:T2)
        n706 = Equal?(x=w979, y=3) -> (x = y?=w975:bool)
        n707 = Not(x=w975) -> (.not. x?=w974:bool)
        n708 = And(x=w980, y=w975) -> (x .and. y?=w977:T7)
        n709 = local write "commu"(w974) -> ()
        n710 = Select(t=w978, s=w977, f=w976) -> (s? t:f=w973:T2)
      }
      frame "TAB 3" {
        n711 = local read "Index ที่มากที่สุด"() -> (w990:i32)
        n712 = local read "call_back"() -> (w987:bool)
        n713 = Subtract(x=w985, y=2) -> (x-y=w983:u32)
        n714 = Equal?(x=w990, y=3) -> (x = y?=w988:bool)
        n715 = And(x=w987, y=w988) -> (x .and. y?=w989:bool)
        n716 = Not(x=w988) -> (.not. x?=w986:bool)
        n717 = local write "call"(w986) -> ()
        n718 = Select(t=w983, s=w989, f=w985) -> (s? t:f=w982:u32)
      }
      frame "TAB 4" {
        n719 = local read "Index ที่มากที่สุด"() -> (w1000:i32)
        n720 = local read "BACK_Page4"() -> (w997:bool)
        n721 = Subtract(x=w994, y=3) -> (x-y=w993:u32)
        n722 = Equal?(x=w1000, y=3) -> (x = y?=w998:bool)
        n723 = And(x=w997, y=w998) -> (x .and. y?=w999:bool)
        n724 = Not(x=w998) -> (.not. x?=w996:bool)
        n725 = local write "ele"(w996) -> ()
        n726 = Select(t=w993, s=w999, f=w994) -> (s? t:f=w992:u32)
      }
      frame "TAB 5" {
        n727 = local read "BACK_Page5"() -> (w1004:bool)
        n728 = local read "Index ที่มากที่สุด"() -> (w1010:i32)
        n729 = Subtract(x=w1006, y=3) -> (x-y=w1005:u32)
        n730 = Equal?(x=w1010, y=3) -> (x = y?=w1008:bool)
        n731 = And(x=w1004, y=w1008) -> (x .and. y?=w1009:bool)
        n732 = Not(x=w1008) -> (.not. x?=w1003:bool)
        n733 = local write "Emotion"(w1003) -> ()
        n734 = Select(t=w1005, s=w1009, f=w1006) -> (s? t:f=w1002:u32)
      }
      frame "TAB 6" {
        n735 = local read "BACK_Page6"() -> (w1014:T9)
        n736 = local read "Index ที่มากที่สุด"() -> (w1020:i32)
        n737 = Subtract(x=w1016, y=4) -> (x-y=w1015:u32)
        n738 = Equal?(x=w1020, y=3) -> (x = y?=w1018:bool)
        n739 = And(x=w1014, y=w1018) -> (x .and. y?=w1019:T9)
        n740 = Not(x=w1018) -> (.not. x?=w1013:bool)
        n741 = local write "Activity"(w1013) -> ()
        n742 = Select(t=w1015, s=w1019, f=w1016) -> (s? t:f=w1012:u32)
      }
      frame "TAB 7" {
        n743 = local read "BACK_Page7"() -> (w1024:bool)
        n744 = local read "Index ที่มากที่สุด"() -> (w1030:i32)
        n745 = Subtract(x=w1026, y=4) -> (x-y=w1025:u32)
        n746 = Equal?(x=w1030, y=3) -> (x = y?=w1028:bool)
        n747 = And(x=w1024, y=w1028) -> (x .and. y?=w1029:bool)
        n748 = Not(x=w1028) -> (.not. x?=w1023:bool)
        n749 = local write "ACC"(w1023) -> ()
        n750 = Select(t=w1025, s=w1029, f=w1026) -> (s? t:f=w1022:u32)
      }
    }
    n751 = local write "Tab Control"(w944) -> ()
    n752 = Send Notification(notification=w944, notifier=w948, error in (no error)=w946) -> (notifier out=w947:refnum<notifier>, error out=w945:errorcluster)
  }
  n753 = while {
    shift-right: [w1032] -> _
    shift-left: "" -> [w1034]
    stop <- FALSE stop-if-true
    n754 = event shown="[2] \"Text3\": Value Change" {
      selector: _ -> [_ _ _ _]
      dyn-events: _ -> [_ _ _ _]
      timeout: _ -> [_ _ _ _]
      tunnel: w1034 -> [_ _ _ w1039]
      tunnel: ["Massage Send 2" "Massage Send 2" "Massage Send 3" w1038] -> w1032
      event "Text1": Value Change {
        n755 = event-data() -> ()  [unwired: 1 in, 6 out]
      }
      event Value Change {
        n756 = event-data() -> ()  [unwired: 1 in, 6 out]
      }
      event Value Change {
        n757 = event-data() -> ()  [unwired: 1 in, 6 out]
      }
      event "Clearpage 2": Value Change {
        n758 = event-data() -> ("CtlRef"=w1041:refnum<vi>)  [unwired: 1 in, 3 out]
        n759 = property class="Bool (strict)"(reference=w1041) -> ("Label.Text"=w1040:string)  [unwired: 1 in, 2 out]
        n760 = case shown="\"Backspacepage 2\", Default" w1040 {
          tunnel: w1039 -> [w1043 _]
          tunnel: [w1042 ""] -> w1038
          frame "Backspacepage 2", Default {
            n761 = String Length(string=w1043) -> (length=w1044:i32)
            n762 = Decrement(x=w1044) -> (x-1=w1045:i32)
            n763 = String Subset(string=w1043, length (rest)=w1045) -> (substring=w1042:string)  [unwired: 1 in]
          }
          frame "Clearpage 2" {
          }
        }
      }
    }
    "Message Display" <- w1032
  }
  n764 = Release Notifier(notifier=w5, error in (no error)=w3) -> ()  [unwired: 1 in, 3 out]
  n765 = call <vilib>:"Draw Flattened Pixmap.vi"() -> ()  [unwired: 9 in, 1 out]
  n766 = call <vilib>:"Draw Flattened Pixmap.vi"() -> ()  [unwired: 9 in, 1 out]
  n767 = call <vilib>:"Draw Flattened Pixmap.vi"() -> ()  [unwired: 9 in, 1 out]
